vi "Autopatch-v2.1.vi"() -> ()   [LabVIEW 2016]
uses:
  <vilib>/userdefined/High Color/IMAQdx.ctl
  <vilib>/DAQmx/write.llb/DAQmx Write (Analog DBL 1Chan 1Samp).vi
  <vilib>/DAQmx/write.llb/DAQmx Write (Analog Wfm 1Chan NSamp).vi
  <vilib>/DAQmx/read.llb/DAQmx Read (Analog Wfm 1Chan NSamp).vi
  <vilib>/Analysis/baseanly.llb/Mean (DBL).vi
  <vilib>/DAQmx/create/channels.llb/DAQmx Create Channel (AO-Voltage-Basic).vi
  <vilib>/DAQmx/miscellaneous.llb/DAQmx Fill In Error Info.vi
  <vilib>/DAQmx/create/channels.llb/DAQmx Create Channel (AI-Voltage-Basic).vi
  <vilib>/DAQmx/configure/timing.llb/DAQmx Timing (Sample Clock).vi
  <vilib>/DAQmx/configure/trigger.llb/DAQmx Start Trigger (Digital Edge).vi
  <vilib>/Waveform/WDTOps.llb/WDT Waveform Duration DBL.vi
  <vilib>/addons/control/pid/pid.llb/PID (DBL).vi
  <vilib>/vision/driver/NI_Vision_Acquisition_Software.lvlib
  <resource>/objmgr/daqmx.rc
  <vilib>/Analysis/NI_AALBase.lvlib
  <vilib>/measure/NI_MABase.lvlib
  <vilib>/vision/NI_Vision_Development_Module.lvlib
  <vilib>/addons/control/pid/NI_PID_pid.lvlib
  vs/cell/Debug/cell.dll
panel:
  in  "下降/向右":bool
  in  "down":bool
  in  "up":bool
  out "读取缓冲区":string
  in  "调焦步伐/um":i64(ring)=3 items=["1", "10", "100", "1000", "10000"]
  in  "停止运动":bool
  in  "设置移动步长":bool
  in  "返回Z轴坐标":bool
  out "x*y":dbl
  out "电阻值":dbl
  in  "钳制电位":i16(ring) items=["0mv", "-70mv"]
  out "数值":dbl
  in  "自动破膜":bool
  in  "控制箱刺激ON\n/放大器刺激":bool=TRUE
  out "cout":i32
  out "Image 3":T1(plugin-control)
  out "Image 2":T1(plugin-control)
  in  "对比图":bool
  in  "自动封接":bool
  in  "保存数据":bool
  out "是否匹配到？":bool
  in  "PID gains":T2={"proportional gain (Kc)"=-0.05, "integral time (Ti, min)"=0.0, "derivative time (Td, min)"=0.0} caption="PID增益" {"derivative time (Td, min)" format="%.3f"; "integral time (Ti, min)" format="%.3f"; "proportional gain (Kc)" format="%.3f"}
  in  "PID gains 2":T2={"proportional gain (Kc)"=0.05, "integral time (Ti, min)"=0.0, "derivative time (Td, min)"=0.0} caption="PID增益" {"derivative time (Td, min)" format="%.3f"; "integral time (Ti, min)" format="%.3f"; "proportional gain (Kc)" format="%.3f"}
  out "x+y 2":i16
  out "调焦值2":dbl
  out "调焦值 3":dbl
  out "调焦值 4":dbl
  out "变量":dbl
  out "布尔":bool
  in  "聚焦值数组":dbl[](array[numeric])
  in  "下降步伐/um":dbl=1.0
  in  "自动接触":bool
  out "清晰度评价函数":dbl(graph)
  in  "针尖自动移动":bool
  in  "针尖细对焦":bool
  in  "针尖粗对焦":bool
  out "二值化":T1(plugin-control)
  in  "Range":cluster{"Lower value":sgl, "Upper value":sgl}={"Lower value"=0.0, "Upper value"=150.0} {"Upper value" format="%.2f"; "Lower value" format="%.2f"}
  in  "Operation":T3(ring)=enum."Dilate"
  in  "Number of Erosion":i32=10
  out "Particle Reports (Pixels)":T4(array[cluster]) {"Orientation" format="%.2f"; "Dimensions"."Height" format="%.2f"; "Dimensions"."Width" format="%.2f"; "Center of Mass"."Y" format="%.2f"; "Center of Mass"."X" format="%.2f"; "Bounding Rect"."Bottom" format="%.2f"; "Bounding Rect"."Right" format="%.2f"; "Bounding Rect"."Top" format="%.2f"; "Bounding Rect"."Left" format="%.2f"; "Number of Holes" format="%.2f"; "Area" format="%.2f"}
  out "Right":dbl
  out "目标坐标":i32[](array[numeric])
  in  "针尖模板匹配":bool=TRUE
  in  "基路径":path=path "E:/膜片/膜片钳/程序/CCD/模板40倍.jpg"
  out "Number of Matches":i32
  in  "Minimum Contrast":i32 min=0 max=255 step=1
  in  "Minimum Match Score":sgl=650.0 min=0 max=1000 format="%.2f"
  in  "Number of Matches Requested":i32=1 min=1
  out "Matches 2":T5(array[cluster]) {"Bounding Box"."y" format="%.2f"; "Bounding Box"."x" format="%.2f"; "Position"."y" format="%.2f"; "Position"."x" format="%.2f"; "Score" format="%.2f"; "Scale" format="%.2f"; "Angle" format="%.2f"}
  in  "Match Mode":u16(ring) items=["Shift Invariant", "Rotation Invariant"]
  out "针尖坐标":sgl[](array[numeric])
  in  "入液阻值校准":bool
  out "校准的入液阻值":dbl
  out "错误输出 3":errorcluster caption="错误输出"
  in  "低负开关":bool
  in  "低正开关":bool
  in  "大气压":bool
  in  "高负开关":bool
  in  "高正开关":bool
  in  "case":dbl
  out "测量值":dbl
  out "给定值":dbl
  out "输出气压波形图表":cluster{dbl, "低负":dbl}(graph)
  in  "低负":sgl(knob)=-0.45548448
  in  "高负":sgl(knob)=-5.0
  in  "低正":sgl(knob)=0.49642125 scale=0.0..2.0
  in  "高正":sgl(knob)=10.718505 scale=0.0..15.0
  in  "采样率":u32=255
  in  "DevIndex":i32
  in  "Holding Voltage":dbl=-70.0
  out "Negative Peak":dbl
  out "阻值波形图表":dbl(graph)
  out "Resistance(MΩ)":dbl
  out "！":bool
  in  "下拉列表":u16(ring) items=["Voltage Clamp", "Current Clamp"]
  out "电流信号波形图":waveform(dbl)(graph)
  in  "frequency":dbl=20.0
  in  "Averaging":i32=5
  in  "amplitude":dbl=0.01
  in  "阻值数组":dbl[](array[numeric])
  out "循环时间":u32
  out "Image":T1(plugin-control)
  out "错误输出":errorcluster
  in  "停止":bool
  in  "Session In":T6="cam1"
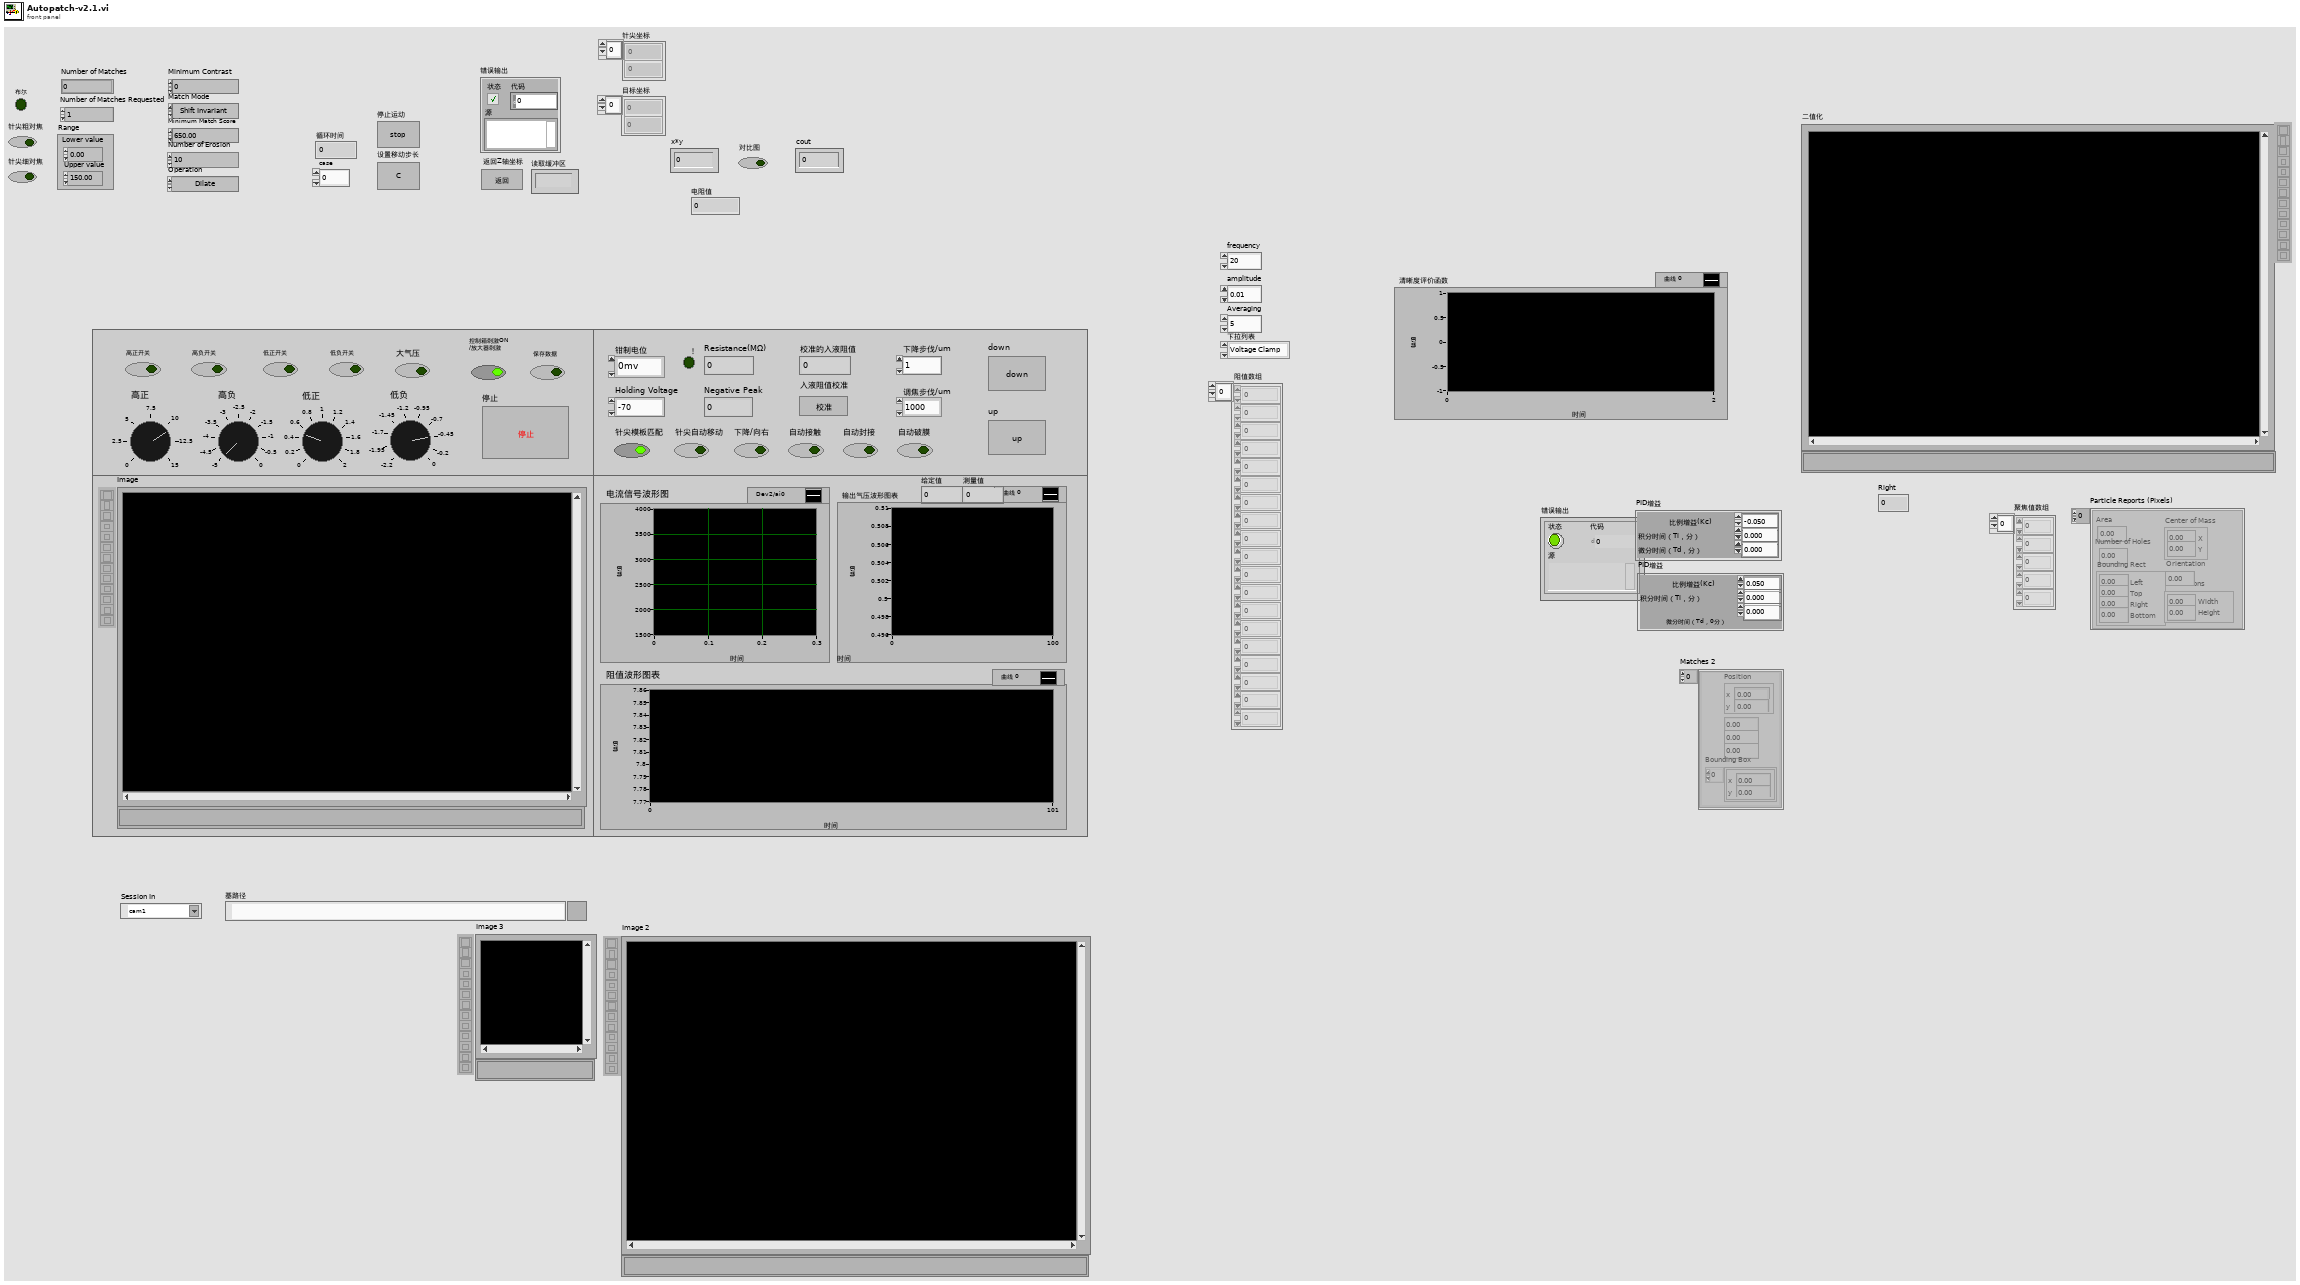
[diagram p1: front panel]
types:
  T1 = typedef "IMAQ Image.ctl" = refnum<image>
  T2 = cluster{"proportional gain (Kc)":dbl, "integral time (Ti, min)":dbl, "derivative time (Td, min)":dbl}
  T3 = enum32{"AutoM", "Close", "Dilate", "Erode", "Gradient", "Gradient out", "Gradient in", "Hit miss", "Open", "PClose", "POpen", "Thick", "Thin"}
  T4 = cluster{"Area":dbl, "Number of Holes":dbl, "Bounding Rect":cluster{"Left":dbl, "Top":dbl, "Right":dbl, "Bottom":dbl}, "Center of Mass":cluster{"X":dbl, "Y":dbl}, "Orientation":dbl, "Dimensions":cluster{"Width":dbl, "Height":dbl}}[]
  T5 = cluster{"Position":cluster{"x":sgl, "y":sgl}, "Angle":sgl, "Scale":sgl, "Score":sgl, "Bounding Box":cluster{"x":sgl, "y":sgl}[]}[]
  T6 = typedef "IMAQdx.ctl" = refnum<k21>
  T7 = enum16{"open", "replace", "create", "open or create", "replace or create", "replace or create with confirmation"}
  T8 = typedef "Image Type" = u32
  T9 = cluster{"Averaging":i32, "frequency":dbl, "amplitude":dbl, "Proportion":dbl, "Fs":dbl}
  T10 = enum16{"Sine Wave", "Triangle Wave", "Square Wave", "Sawtooth Wave"}
  T11 = cluster{"Global Rectangle":i32[], "Contours":cluster{"Contour Type":u32, "ROI Type":u32, "Points":i32[]}[]}
  T12 = cluster{"Position":cluster{"x":sgl, "y":sgl}, "Angle":sgl, "Scale":sgl, "Score":sgl, "Bounding Box":cluster{"x":sgl, "y":sgl}[]}
  T13 = cluster{"Area":dbl, "Number of Holes":dbl, "Bounding Rect":cluster{"Left":dbl, "Top":dbl, "Right":dbl, "Bottom":dbl}, "Center of Mass":cluster{"X":dbl, "Y":dbl}, "Orientation":dbl, "Dimensions":cluster{"Width":dbl, "Height":dbl}}
  T14 = cluster{"Left":dbl, "Top":dbl, "Right":dbl, "Bottom":dbl}
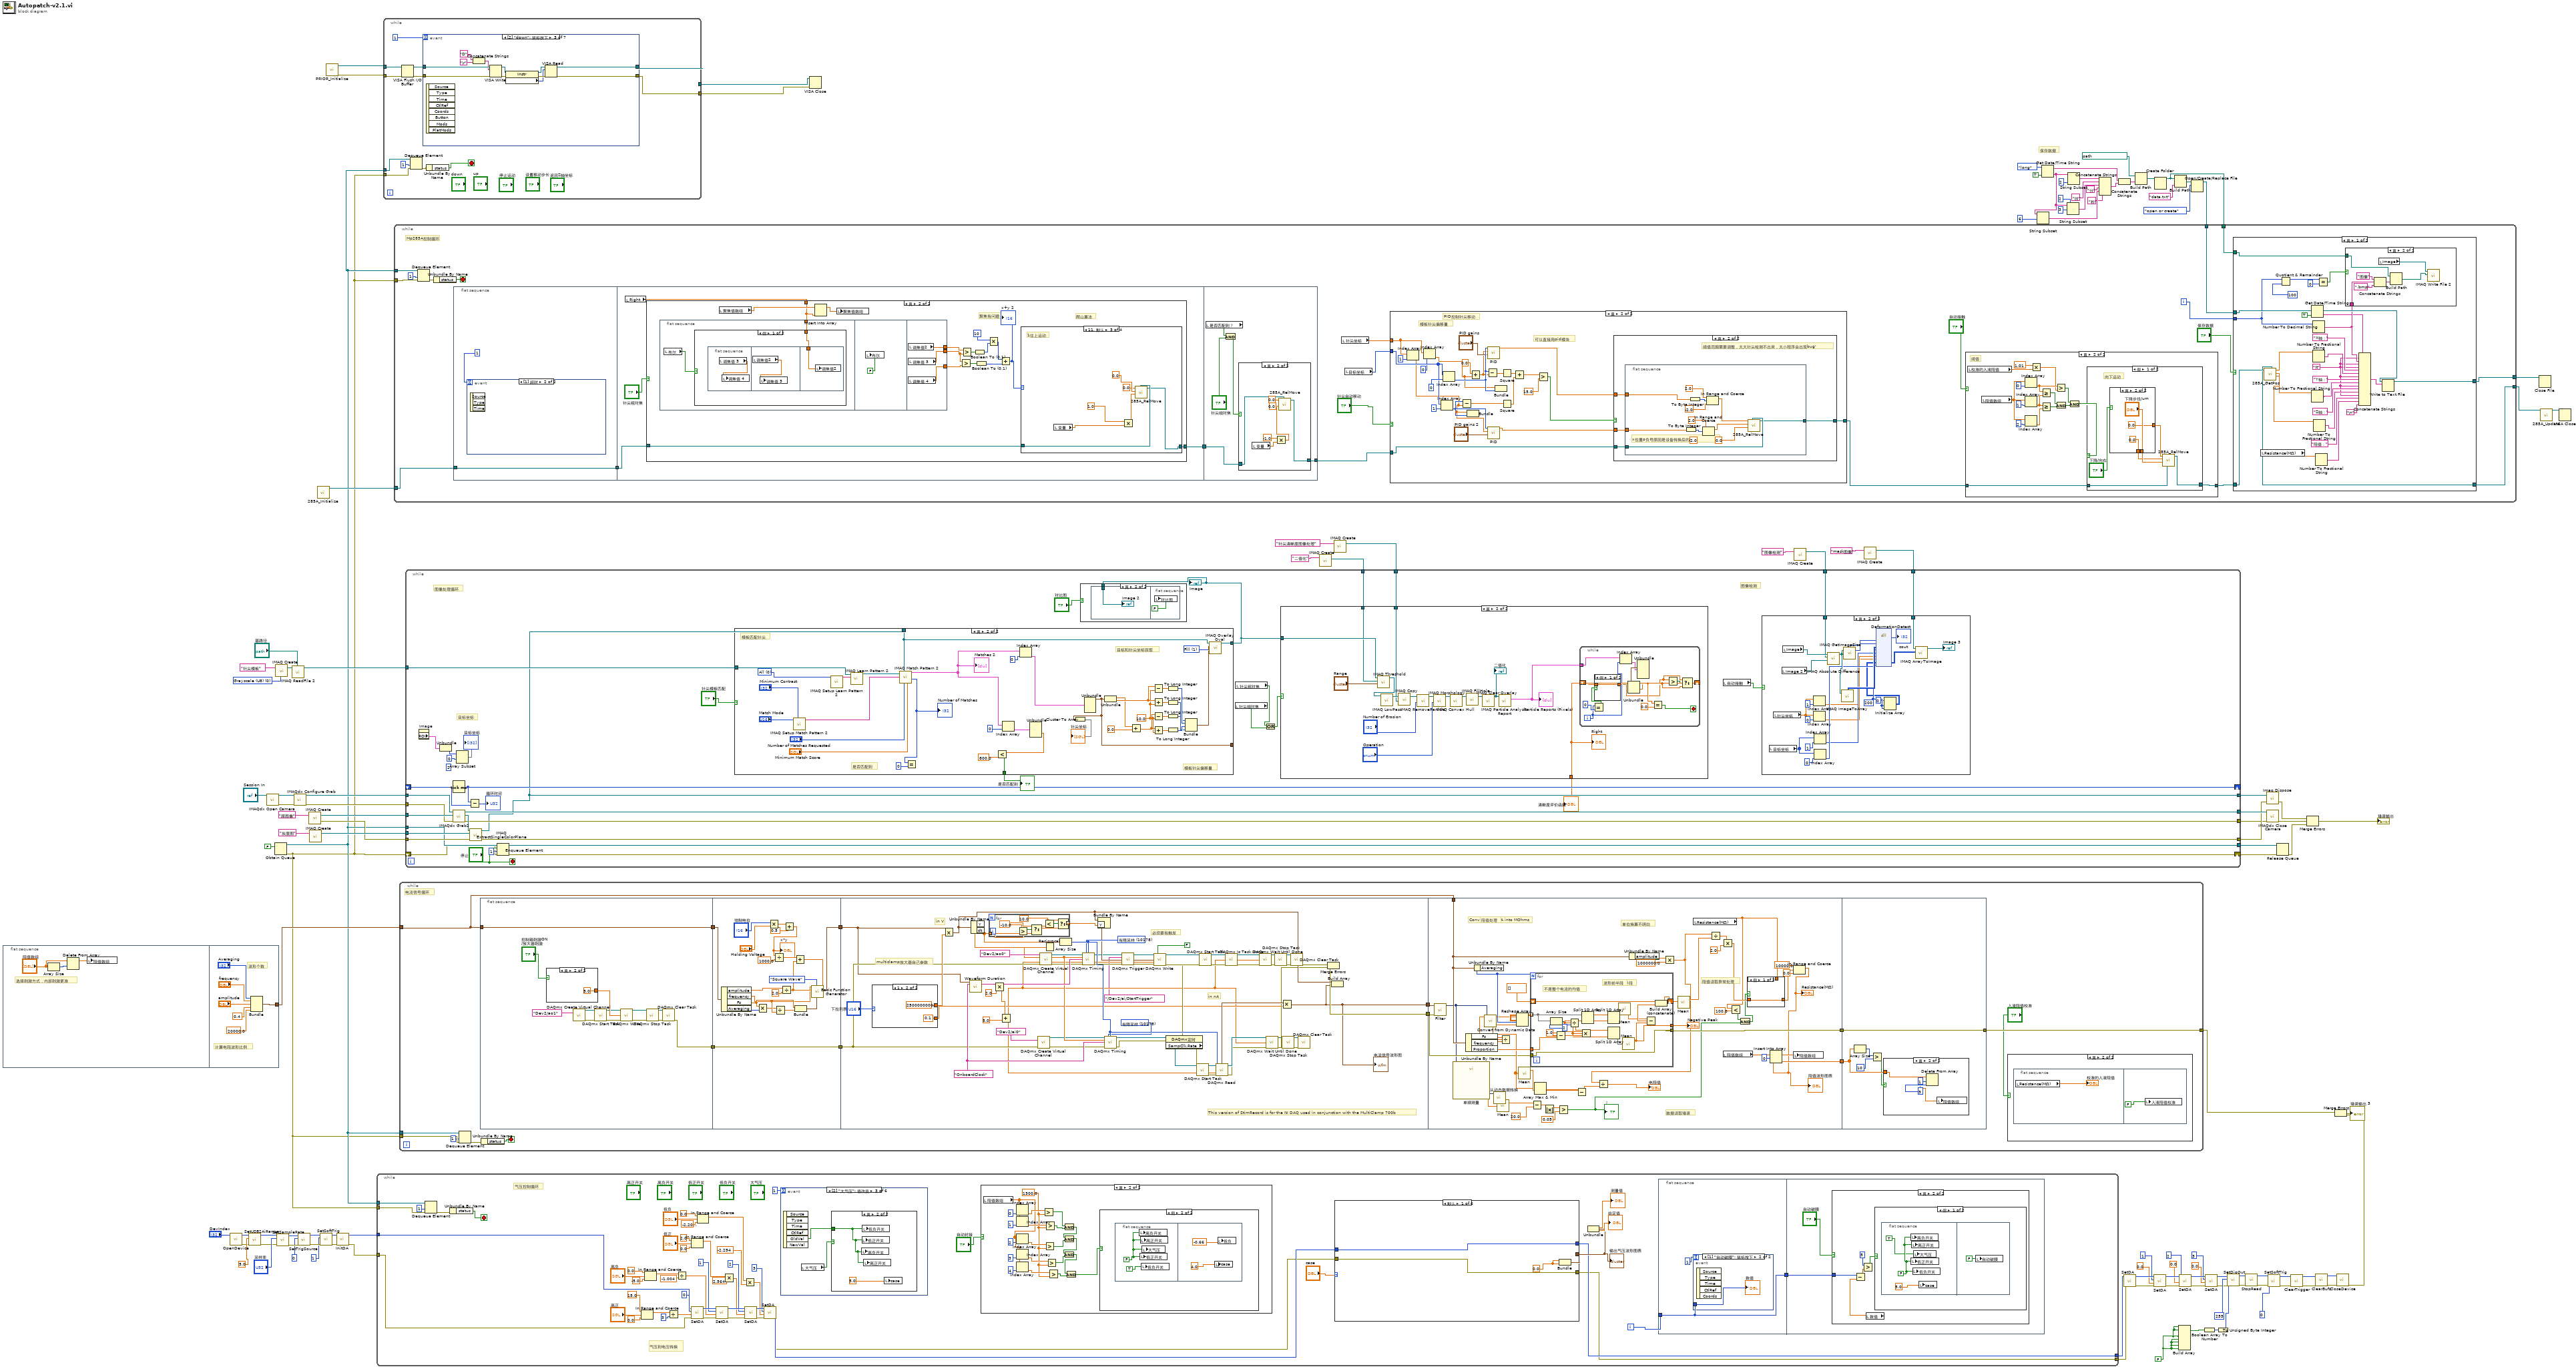
[diagram p0: block diagram]
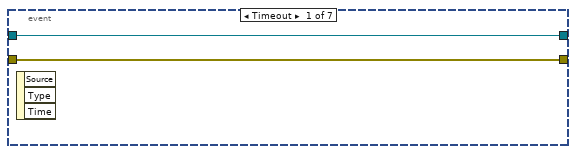
[diagram p2: hidden frame]
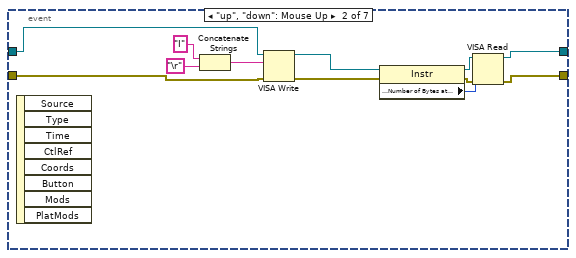
[diagram p3: hidden frame]
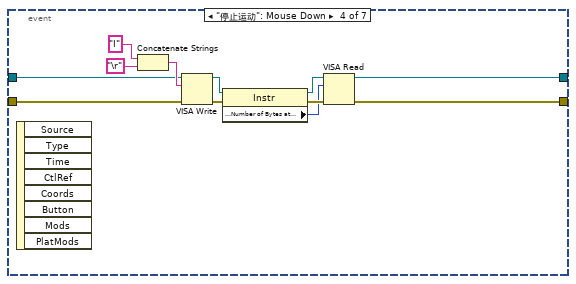
[diagram p4: hidden frame]
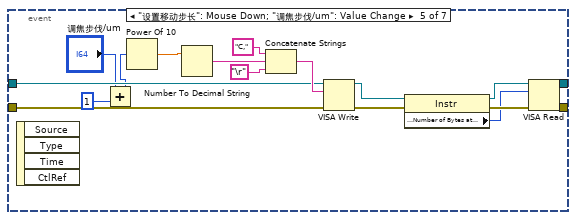
[diagram p5: hidden frame]
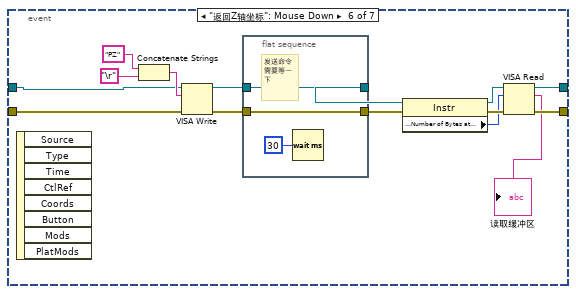
[diagram p6: hidden frame]
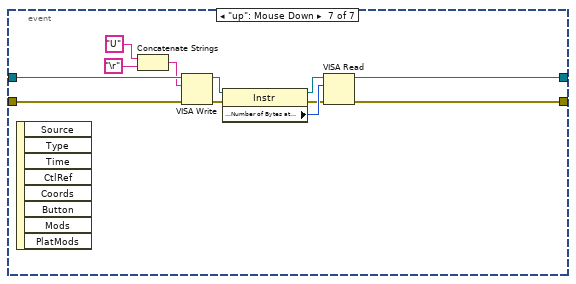
[diagram p7: hidden frame]
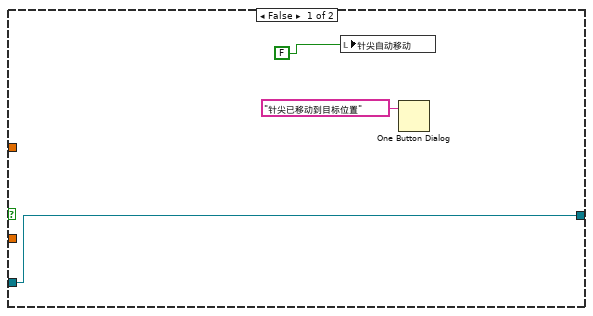
[diagram p11: hidden frame]
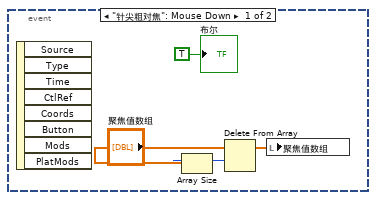
[diagram p12: hidden frame]
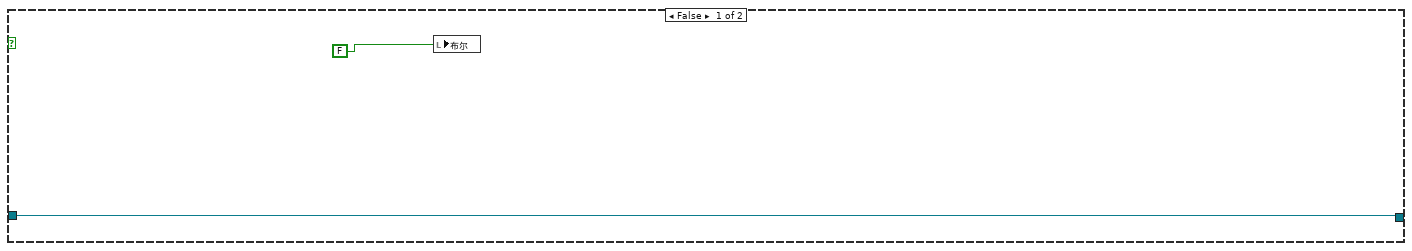
[diagram p13: hidden frame]
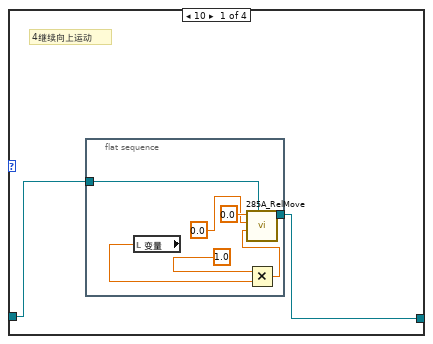
[diagram p14: hidden frame]
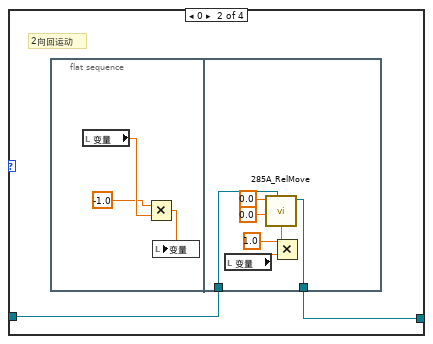
[diagram p15: hidden frame]
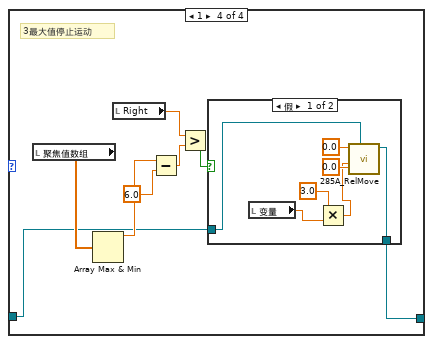
[diagram p16: hidden frame]
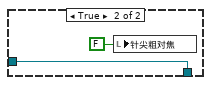
[diagram p17: hidden frame]
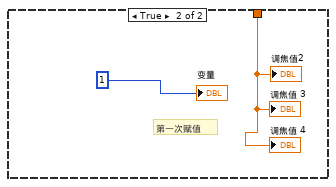
[diagram p18: hidden frame]
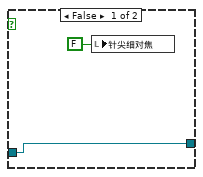
[diagram p19: hidden frame]
diagram:
  w47 = T8 0 items=["Grayscale (U8)", "Grayscale (I16)", "Grayscale (SGL)", "Complex (CSG)", "RGB (U32)", "HSL (U32)", "RGB (U64)", "Grayscale (U16)"] ("Image Type")
  w61 = FALSE
  # "保存数据"
  n1 = flat-sequence {
    tunnel: [w124] -> w108
    frame #0 {
      # "选择刺激方式，内部刺激更准"
      n2 = Array Size(array="阻值数组") -> (size(s)=w123:i32)
      n3 = Delete From Array(array="阻值数组", length=w123) -> (array with subset deleted=w121:dbl[])  [unwired: 1 in, 1 out]
      n4 = local write "阻值数组"(w121) -> ()
    }
    frame #1 {
      # "波形个数"
      # "计算电阻波形比例"
      n5 = Bundle("Averaging"="Averaging", "frequency"="frequency", "amplitude"="amplitude", "Proportion"=0.4, "Fs"=20000.0) -> (w124:T9)  [unwired: 1 in]
    }
  }
  n6 = call "OpenDevice.vi"("DevIndex"="DevIndex") -> ("错误输出"=w88:errorcluster, "DevIndex Output"=w86:i32)  [unwired: 9 in]
  n7 = call "SetUSB2AiRange.vi"("错误输入（无错误）"=w88, "Range"=sgl 5.0, "DevIndex"=w86) -> ("错误输出"=w97:errorcluster, "DevIndex Output"=w95:i32)  [unwired: 7 in]
  n8 = call <vilib>:"IMAQdx Open Camera.vi"("Session In"="Session In") -> ("error out"=w120:errorcluster, "Session Out"=w117:T6)  [unwired: 9 in]
  n9 = Obtain Queue(element data type=FALSE) -> (queue out=w2:refnum<queue>, error out=w1:errorcluster)  [unwired: 4 in, 1 out]
  n10 = call "IMAQ Create"("Image Name"="针尖模板", "Image Type"=w47) -> ("New Image"=w48:T1)  [unwired: 3 in, 1 out]
  n11 = call "SetSampleRate.vi"("错误输入（无错误）"=w97, "SampleRate"="采样率", "DevIndex"=w95) -> ("错误输出"=w98:errorcluster, "DevIndex Output"=w96:i32)  [unwired: 7 in]
  n12 = call "IMAQ ReadFile 2"("File Path"="基路径", "Image"=w48) -> ("Image Out"=w46:T1)  [unwired: 5 in, 4 out]
  n13 = call <vilib>:"IMAQdx Configure Grab.vi"("error in"=w120, "Session In"=w117) -> ("error out"=w105:errorcluster, "Session Out"=w118:T6)  [unwired: 8 in]
  n14 = call "SetTrigSource.vi"("错误输入（无错误）"=w98, "TrigSource"=u8 0, "DevIndex"=w96) -> ("错误输出"=w93:errorcluster, "DevIndex Output"=w92:i32)  [unwired: 7 in]
  n15 = call "IMAQ Create"("Image Name"="原图像") -> ("New Image"=w116:T1, "error out"=w103:errorcluster)  [unwired: 4 in]
  n16 = call "IMAQ Create"("Image Name"="灰度图") -> ("New Image"=w109:T1)  [unwired: 4 in, 1 out]
  n17 = call "285A_Initialize.vi"() -> ("VISA资源名称输出"=w41:refnum<visa-resource-name>)  [unwired: 10 in, 1 out]
  n18 = call "SetSoftTrig.vi"("错误输入（无错误）"=w93, "Trig"=u8 1, "DevIndex"=w92) -> ("错误输出"=w89:errorcluster, "DevIndex Output"=w87:i32)  [unwired: 7 in]
  n19 = call "PRIOR_Initialize.vi"() -> ("错误输出"=w5:errorcluster, "VISA资源名称输出"=w6:refnum<visa-resource-name>)  [unwired: 10 in]
  n20 = call "InitDA.vi"("错误输入（无错误）"=w89, "DevIndex"=w87) -> ("错误输出"=w83:errorcluster, "DevIndex Output"=w84:i32)  [unwired: 8 in]
  n21 = while {
    tunnel: w84 -> [w143]
    tunnel: w2 -> [w182]
    tunnel: w1 -> [w181]
    tunnel: [w135] -> w8
    tunnel: w83 -> [w142]
    tunnel: [w133] -> w7
    i -> [w131]
    stop <- w178 stop-if-true
    # "气压控制循环"
    # "气压到电压转换"
    n22 = Dequeue Element(queue=w182, timeout in ms (-1)=1 ("超时毫秒(-1)"), error in (no error)=w181) -> (error out=w179:errorcluster)  [unwired: 3 out]
    n23 = Unbundle By Name(w179) -> ("status"=w178:bool)
    n24 = In Range and Coerce(upper limit=sgl 15.0 ("上限"), x="高正", lower limit=sgl 0.0 ("下限")) -> (coerced(x)=w146:sgl)  [unwired: 1 out]
    n25 = In Range and Coerce(upper limit=sgl 0.0 ("上限"), x="高负", lower limit=sgl -5.0 ("下限")) -> (coerced(x)=w150:sgl)  [unwired: 1 out]
    n26 = Divide(x=w146, y=3) -> (x/y=w167:sgl)
    n27 = Divide(x=w150, y=-1.004) -> (x/y=w163:dbl)
    n28 = In Range and Coerce(upper limit=sgl 2.0 ("上限"), x="低正", lower limit=sgl 0.0 ("下限")) -> (coerced(x)=w154:sgl)  [unwired: 1 out]
    n29 = call "SetDA.vi"("错误输入（无错误）"=w142, "DAVolt"=w167, "DANum"=u8 0, "DevIndex"=w143) -> ("错误输出"=w176:errorcluster, "DevIndex Output"=w177:i32)  [unwired: 6 in]
    n30 = In Range and Coerce(upper limit=sgl 0.0 ("上限"), x="低负", lower limit=sgl -2.2 ("下限")) -> (coerced(x)=w156:sgl)  [unwired: 1 out]
    n31 = call "SetDA.vi"("错误输入（无错误）"=w176, "DAVolt"=w163, "DANum"=u8 1, "DevIndex"=w177) -> ("错误输出"=w175:errorcluster, "DevIndex Output"=w174:i32)  [unwired: 6 in]
    n32 = Multiply(x=w154, y=2.564) -> (x*y=w160:dbl)
    n33 = Multiply(x=w156, y=-2.294) -> (x*y=w161:dbl)
    n34 = call "SetDA.vi"("错误输入（无错误）"=w175, "DAVolt"=w160, "DANum"=u8 2, "DevIndex"=w174) -> ("错误输出"=w172:errorcluster, "DevIndex Output"=w173:i32)  [unwired: 6 in]
    n35 = call "SetDA.vi"("错误输入（无错误）"=w172, "DAVolt"=w161, "DANum"=u8 3, "DevIndex"=w173) -> ("错误输出"=w136:errorcluster, "DevIndex Output"=w137:i32)  [unwired: 6 in]
    n36 = event shown="[2] \"大气压\": 值改变" {
      selector: _ -> [_ _ _ _ _ _]
      dyn-events: _ -> [_ _ _ _ _ _]
      timeout: 1 -> [_ _ _ _ _ _]
      event "高正开关": Value Change {
        n37 = event-data() -> ("OldVal"=w231:bool)  [unwired: 1 in, 5 out]
        n38 = local read "高正开关"() -> (w232:bool)
        n39 = case shown="真" w232 {
          tunnel: w231 -> [_ w234]
          frame False {
          }
          frame True {
            n40 = local write "高负开关"(w234) -> ()
            n41 = local write "低负开关"(w234) -> ()
            n42 = local write "低正开关"(w234) -> ()
            n43 = local write "大气压"(w234) -> ()
            n44 = local write "case"(1.0) -> ()
          }
        }
      }
      event Timeout {
        n45 = event-data() -> ()  [unwired: 1 in, 3 out]
      }
      event "大气压": Value Change {
        n46 = event-data() -> ("OldVal"=w235:bool)  [unwired: 1 in, 5 out]
        n47 = local read "大气压"() -> (w236:bool)
        n48 = case shown="真" w236 {
          tunnel: w235 -> [_ w238]
          frame False {
          }
          frame True {
            n49 = local write "高负开关"(w238) -> ()
            n50 = local write "低正开关"(w238) -> ()
            n51 = local write "低负开关"(w238) -> ()
            n52 = local write "高正开关"(w238) -> ()
            n53 = local write "case"(5.0) -> ()
          }
        }
      }
      event "低正开关": Value Change {
        n54 = event-data() -> ("OldVal"=w240:bool)  [unwired: 1 in, 5 out]
        n55 = local read "低正开关"() -> (w239:bool)
        n56 = case shown="真" w239 {
          tunnel: w240 -> [_ w242]
          frame False {
          }
          frame True {
            n57 = local write "高正开关"(w242) -> ()
            n58 = local write "高负开关"(w242) -> ()
            n59 = local write "低负开关"(w242) -> ()
            n60 = local write "大气压"(w242) -> ()
            n61 = local write "case"(3.0) -> ()
          }
        }
      }
      event "低负开关": Value Change {
        n62 = event-data() -> ("OldVal"=w244:bool)  [unwired: 1 in, 5 out]
        n63 = local read "低负开关"() -> (w243:bool)
        n64 = case shown="真" w243 {
          tunnel: w244 -> [_ w246]
          frame False {
          }
          frame True {
            n65 = local write "高负开关"(w246) -> ()
            n66 = local write "低正开关"(w246) -> ()
            n67 = local write "高正开关"(w246) -> ()
            n68 = local write "大气压"(w246) -> ()
            n69 = local write "case"(4.0) -> ()
          }
        }
      }
      event "高负开关": Value Change {
        n70 = event-data() -> ("OldVal"=w248:bool)  [unwired: 1 in, 5 out]
        n71 = local read "高负开关"() -> (w247:bool)
        n72 = case shown="真" w247 {
          tunnel: w248 -> [_ w250]
          frame False {
          }
          frame True {
            n73 = local write "低正开关"(w250) -> ()
            n74 = local write "低负开关"(w250) -> ()
            n75 = local write "高正开关"(w250) -> ()
            n76 = local write "大气压"(w250) -> ()
            n77 = local write "case"(2.0) -> ()
          }
        }
      }
    }
    n78 = case shown="真" "自动封接" {
      frame False {
      }
      frame True {
        w205 = 1300.0 ("y")
        n79 = local read "阻值数组"() -> (w206:dbl[])
        n80 = Index Array(array=w206, index=0 ("索引")) -> (element=w208:dbl)
        n81 = Index Array(array=w206, index=1 ("索引")) -> (element=w207:dbl)
        n82 = Index Array(array=w206, index=2 ("索引")) -> (element=w216:dbl)
        n83 = Index Array(array=w206, index=3 ("索引")) -> (element=w215:dbl)
        n84 = Index Array(array=w206, index=4 ("索引")) -> (element=w214:dbl)
        n85 = Greater?(x=w208, y=w205) -> (0:w213:bool)
        n86 = Greater?(x=w216, y=w205) -> (0:w211:bool)
        n87 = Greater?(x=w207, y=w205) -> (0:w212:bool)
        n88 = Greater?(x=w215, y=w205) -> (0:w210:bool)
        n89 = Greater?(x=w214, y=w205) -> (0:w209:bool)
        n90 = And(x=w213, y=w212) -> (x .and. y?=w204:bool)
        n91 = And(x=w204, y=w211) -> (x .and. y?=w203:bool)
        n92 = And(x=w203, y=w210) -> (x .and. y?=w202:bool)
        n93 = And(x=w202, y=w209) -> (x .and. y?=w201:bool)
        n94 = case shown="假" w201 {
          frame True {
            n95 = flat-sequence {
              frame #0 {
                w222 = FALSE
                n96 = local write "高负开关"(w222) -> ()
                n97 = local write "低负开关"(w222) -> ()
                n98 = local write "低正开关"(w222) -> ()
                n99 = local write "高正开关"(w222) -> ()
                n100 = local write "大气压"(TRUE) -> ()
              }
              frame #1 {
                n101 = local write "case"(5.0) -> ()
              }
              frame #2 {
                n102 = local write "自动封接"(FALSE) -> ()
                n103 = One Button Dialog(message="已形成G欧封接！" ("消息")) -> ()  [unwired: 1 in, 1 out]
              }
            }
          }
          frame False {
            n104 = flat-sequence {
              frame #0 {
                w227 = FALSE
                n105 = local write "高负开关"(w227) -> ()
                n106 = local write "低正开关"(w227) -> ()
                n107 = local write "高正开关"(w227) -> ()
                n108 = local write "低负开关"(TRUE) -> ()
                n109 = local write "大气压"(w227) -> ()
              }
              frame #1 {
                n110 = local write "case"(4.0) -> ()
                n111 = local write "低负"(-0.66) -> ()
              }
            }
          }
        }
      }
    }
    n112 = case shown="默认" "case" {
      tunnel: w137 -> [w254 w274 w296 w320 w344 w357]
      tunnel: w136 -> [w253 w273 w295 w319 w343 w356]
      tunnel: [w254 w256 w287 w314 w336 w354] -> w135
      tunnel: [w253 w264 w288 w313 w337 w353] -> w133
      tunnel: [w251 w255 w279 w303 w327 w351] -> w139
      frame Default {
        w252 = 0.0
        n113 = Bundle(w252, w252) -> (w251:cluster{dbl, dbl})  [unwired: 1 in]
      }
      frame 1 {
        w271 = TRUE
        w272 = FALSE
        n114 = Build Array(w272, w271, w271, w272, w272, w272, w272, w272) -> (w275:bool[])
        n115 = Boolean Array To Number(Boolean array=w275) -> (number=w278:u32)
        n116 = To Unsigned Byte Integer(number=w278) -> (unsigned 8bit integer=w277:u8)
        n117 = call "StartRead.vi"("错误输入（无错误）"=w273, "DevIndex"=w274) -> ("错误输出"=w269:errorcluster, "DevIndex Output"=w270:i32)  [unwired: 8 in]
        n118 = call "SetDioOut.vi"("错误输入（无错误）"=w269, "DioOut"=w277, "DioChanSel"=u8 255, "DevIndex"=w270) -> ("错误输出"=w265:errorcluster, "DevIndex Output"=w266:i32)  [unwired: 6 in]
        n119 = call "GetAiChans.vi"("错误输入（无错误）"=w265, "Num"=u32 1, "ChanSel"=u16 1, "DevIndex"=w266) -> ("错误输出"=w264:errorcluster, "Ai"=w261:sgl[][], "DevIndex Output"=w256:i32)  [unwired: 4 in, 1 out]
        n120 = Index Array(array=w261, index (row)=0, index (col)=0) -> (element=w258:sgl)
        n121 = local read "高正"() -> (w260:sgl)
        n122 = Multiply(x=w258, y=3) -> (x*y=w257:sgl)
        n123 = Bundle(w257, "高正"=w260) -> (w255:cluster{sgl, "高正":sgl})  [unwired: 1 in]
      }
      frame 2 {
        w294 = TRUE
        w293 = FALSE
        n124 = Build Array(w293, w294, w293, w293, w294, w293, w293, w293) -> (w297:bool[])
        n125 = Boolean Array To Number(Boolean array=w297) -> (number=w302:u32)
        n126 = To Unsigned Byte Integer(number=w302) -> (unsigned 8bit integer=w301:u8)
        n127 = call "StartRead.vi"("错误输入（无错误）"=w295, "DevIndex"=w296) -> ("错误输出"=w298:errorcluster, "DevIndex Output"=w299:i32)  [unwired: 8 in]
        n128 = call "SetDioOut.vi"("错误输入（无错误）"=w298, "DioOut"=w301, "DioChanSel"=u8 255, "DevIndex"=w299) -> ("错误输出"=w289:errorcluster, "DevIndex Output"=w290:i32)  [unwired: 6 in]
        n129 = call "GetAiChans.vi"("错误输入（无错误）"=w289, "Num"=u32 1, "ChanSel"=u16 2, "DevIndex"=w290) -> ("错误输出"=w288:errorcluster, "Ai"=w284:sgl[][], "DevIndex Output"=w287:i32)  [unwired: 4 in, 1 out]
        n130 = Unbundle(w289) -> ()  [unwired: 3 out]
        n131 = Index Array(array=w284, index (row)=0, index (col)=0) -> (element=w282:sgl)
        n132 = local read "高负"() -> (w283:sgl)
        n133 = Multiply(x=w282, y=-1.004) -> (x*y=w280:dbl)
        n134 = Bundle(w280, "高负"=w283) -> (w279:cluster{dbl, "高负":sgl})  [unwired: 1 in]
      }
      frame 3 {
        w305 = FALSE
        n135 = Build Array(w305, w305, w305, TRUE, w305, w305, w305, w305) -> (w321:bool[])
        n136 = Boolean Array To Number(Boolean array=w321) -> (number=w326:u32)
        n137 = To Unsigned Byte Integer(number=w326) -> (unsigned 8bit integer=w325:u8)
        n138 = call "StartRead.vi"("错误输入（无错误）"=w319, "DevIndex"=w320) -> ("错误输出"=w322:errorcluster, "DevIndex Output"=w323:i32)  [unwired: 8 in]
        n139 = call "SetDioOut.vi"("错误输入（无错误）"=w322, "DioOut"=w325, "DioChanSel"=u8 255, "DevIndex"=w323) -> ("错误输出"=w315:errorcluster, "DevIndex Output"=w316:i32)  [unwired: 6 in]
        n140 = call "GetAiChans.vi"("错误输入（无错误）"=w315, "Num"=u32 1, "ChanSel"=u16 4, "DevIndex"=w316) -> ("错误输出"=w313:errorcluster, "Ai"=w310:sgl[][], "DevIndex Output"=w314:i32)  [unwired: 4 in, 1 out]
        n141 = Unbundle(w315) -> ()  [unwired: 3 out]
        n142 = Index Array(array=w310, index (row)=0, index (col)=0) -> (element=w308:sgl)
        n143 = local read "低正"() -> (w309:sgl)
        n144 = Divide(x=w308, y=2.564) -> (x/y=w306:dbl)
        n145 = Bundle(w306, "低正"=w309) -> (w303:cluster{dbl, "低正":sgl})  [unwired: 1 in]
      }
      frame 4 {
        w328 = FALSE
        n146 = call "StartRead.vi"("错误输入（无错误）"=w343, "DevIndex"=w344) -> ("错误输出"=w346:errorcluster, "DevIndex Output"=w347:i32)  [unwired: 8 in]
        n147 = local read "低负"() -> (w332:sgl)
        n148 = Build Array(w328, w328, w328, w328, w328, TRUE, w328, w328) -> (w345:bool[])
        n149 = Boolean Array To Number(Boolean array=w345) -> (number=w350:u32)
        n150 = To Unsigned Byte Integer(number=w350) -> (unsigned 8bit integer=w349:u8)
        n151 = call "SetDioOut.vi"("错误输入（无错误）"=w346, "DioOut"=w349, "DioChanSel"=u8 255, "DevIndex"=w347) -> ("错误输出"=w338:errorcluster, "DevIndex Output"=w339:i32)  [unwired: 6 in]
        n152 = Unbundle(w338) -> ()  [unwired: 3 out]
        n153 = call "GetAiChans.vi"("错误输入（无错误）"=w338, "Num"=u32 1, "ChanSel"=u16 8, "DevIndex"=w339) -> ("错误输出"=w337:errorcluster, "Ai"=w333:sgl[][], "DevIndex Output"=w336:i32)  [unwired: 4 in, 1 out]
        n154 = Index Array(array=w333, index (row)=0, index (col)=0) -> (element=w331:sgl)
        n155 = Divide(x=w331, y=-2.294) -> (x/y=w329:dbl)
        n156 = Bundle(w329, "低负"=w332) -> (w327:cluster{dbl, "低负":sgl})  [unwired: 1 in]
      }
      frame 5 {
        w352 = 0.0
        (unwired) TRUE
        w355 = FALSE
        n157 = call "StartRead.vi"("错误输入（无错误）"=w356, "DevIndex"=w357) -> ("错误输出"=w359:errorcluster, "DevIndex Output"=w360:i32)  [unwired: 8 in]
        n158 = Build Array(w355, w355, w355, w355, w355, w355, w355, w355) -> (w358:bool[])
        n159 = Boolean Array To Number(Boolean array=w358) -> (number=w363:u32)
        n160 = To Unsigned Byte Integer(number=w363) -> (unsigned 8bit integer=w362:u8)
        n161 = call "SetDioOut.vi"("错误输入（无错误）"=w359, "DioOut"=w362, "DioChanSel"=u8 255, "DevIndex"=w360) -> ("错误输出"=w353:errorcluster, "DevIndex Output"=w354:i32)  [unwired: 6 in]
        n162 = Unbundle(w353) -> ()  [unwired: 3 out]
        n163 = Bundle(w352, w352) -> (w351:cluster{dbl, dbl})  [unwired: 1 in]
      }
    }
    "输出气压波形图表" <- w139
    n164 = Unbundle(w139) -> (→"测量值":dbl, "高正"=→"给定值":dbl)
    n165 = flat-sequence {
      tunnel: w131 -> [w183]
      tunnel: [w183] -> w130
      tunnel: w130 -> [w186]
      frame #0 {
        n166 = event shown="[1] \"自动破膜\": 鼠标按下" {
          selector: _ -> [_ _]
          dyn-events: _ -> [_ _]
          timeout: 1 -> [_ _]
          tunnel: w183 -> [_ w185]
          event Timeout {
            n167 = event-data() -> ()  [unwired: 1 in, 3 out]
          }
          event "自动破膜": Mouse Down {
            n168 = event-data() -> ()  [unwired: 1 in, 5 out]
            "数值" <- w185
          }
        }
      }
      frame #1 {
        n169 = case shown="真" "自动破膜" {
          tunnel: w186 -> [_ w188]
          frame False {
          }
          frame True {
            n170 = local read "数值"() -> (w192:dbl)
            n171 = Subtract(x=w188, y=w192) -> (x-y=w190:dbl)
            n172 = Greater?(x=5, y=w190) -> (0:w191:bool)
            n173 = case shown="假" w191 {
              frame False {
                n174 = flat-sequence {
                  frame #0 {
                    w195 = FALSE
                    n175 = local write "高负开关"(w195) -> ()
                    n176 = local write "低正开关"(w195) -> ()
                    n177 = local write "高正开关"(w195) -> ()
                    n178 = local write "低负开关"(w195) -> ()
                    n179 = local write "大气压"(TRUE) -> ()
                    n180 = local write "case"(5.0) -> ()
                  }
                  frame #1 {
                    n181 = local write "自动破膜"(FALSE ("自动破膜")) -> ()
                  }
                }
              }
              frame True {
                n182 = flat-sequence {
                  frame #0 {
                    w199 = FALSE
                    n183 = local write "高负开关"(TRUE) -> ()
                    n184 = local write "低正开关"(w199) -> ()
                    n185 = local write "高正开关"(w199) -> ()
                    n186 = local write "低负开关"(w199) -> ()
                    n187 = local write "大气压"(w199) -> ()
                    n188 = local write "case"(2.0) -> ()
                  }
                  frame #1 {
                    n189 = local write "高负"(-5.0) -> ()
                  }
                }
              }
            }
          }
        }
      }
    }
  }
  n190 = while {
    tunnel: w5 -> [w372]
    tunnel: w6 -> [w373]
    tunnel: [w369] -> w3
    tunnel: [w374] -> w4
    tunnel: w2 -> [w366]
    tunnel: w1 -> [w365]
    stop <- w364 stop-if-true
    n191 = VISA Flush I/O Buffer(VISA resource name=w373, error in (no error)=w372) -> (VISA resource name out=w371:refnum<visa-resource-name>, error out=w370:errorcluster)  [unwired: 1 in]
    n192 = Dequeue Element(queue=w366, timeout in ms (-1)=1 ("超时毫秒(-1)"), error in (no error)=w365) -> (error out=w368:errorcluster)  [unwired: 3 out]
    n193 = event shown="[2] \"down\": 鼠标按下" {
      selector: _ -> [_ _ _ _ _ _ _]
      dyn-events: _ -> [_ _ _ _ _ _ _]
      timeout: 1 -> [_ _ _ _ _ _ _]
      tunnel: [w377 w379 w401 w403 w421 w437 w460] -> w374
      tunnel: [w376 w378 w400 w402 w420 w436 w459] -> w369
      tunnel: w371 -> [w377 w381 w399 w405 w423 w439 w458]
      tunnel: w370 -> [w376 w380 w398 w404 w422 w438 w457]
      event Timeout {
        n194 = event-data() -> ()  [unwired: 1 in, 3 out]
      }
      event "up", "down": Mouse Up {
        n195 = event-data() -> ()  [unwired: 1 in, 8 out]
        n196 = Concatenate Strings("I" ("写入缓冲区"), "\r") -> (w389:string)
        n197 = VISA Write ("VISA写入")(VISA resource name=w381, write buffer=w389, error in (no error)=w380) -> (VISA resource name out=w383:refnum<visa-resource-name>, error out=w382:errorcluster)  [unwired: 1 out]
        n198 = property class="Instr"(reference=w383, error in=w382) -> (reference out=w384:refnum<visa-resource-name>, error out=w385:errorcluster, "Serial Settings:Number of Bytes at Serial Port"=w386:u32)
        n199 = VISA Read(VISA resource name=w384, byte count=w386, error in (no error)=w385) -> (VISA resource name out=w379:refnum<visa-resource-name>, error out=w378:errorcluster)  [unwired: 2 out]
      }
      event "down": Mouse Down {
        n200 = event-data() -> ()  [unwired: 1 in, 8 out]
        n201 = Concatenate Strings("D" ("写入缓冲区"), "\r") -> (w390:string)
        n202 = VISA Write ("VISA写入")(VISA resource name=w399, write buffer=w390, error in (no error)=w398) -> (VISA resource name out=w396:refnum<visa-resource-name>, error out=w397:errorcluster)  [unwired: 1 out]
        n203 = property class="Instr"(reference=w396, error in=w397) -> (reference out=w395:refnum<visa-resource-name>, error out=w394:errorcluster, "Serial Settings:Number of Bytes at Serial Port"=w393:u32)
        n204 = VISA Read(VISA resource name=w395, byte count=w393, error in (no error)=w394) -> (VISA resource name out=w401:refnum<visa-resource-name>, error out=w400:errorcluster)  [unwired: 2 out]
      }
      event "停止运动": Mouse Down {
        n205 = event-data() -> ()  [unwired: 1 in, 8 out]
        n206 = Concatenate Strings("I" ("写入缓冲区"), "\r") -> (w406:string)
        n207 = VISA Write ("VISA写入")(VISA resource name=w405, write buffer=w406, error in (no error)=w404) -> (VISA resource name out=w412:refnum<visa-resource-name>, error out=w413:errorcluster)  [unwired: 1 out]
        n208 = property class="Instr"(reference=w412, error in=w413) -> (reference out=w411:refnum<visa-resource-name>, error out=w410:errorcluster, "Serial Settings:Number of Bytes at Serial Port"=w409:u32)
        n209 = VISA Read(VISA resource name=w411, byte count=w409, error in (no error)=w410) -> (VISA resource name out=w403:refnum<visa-resource-name>, error out=w402:errorcluster)  [unwired: 2 out]
      }
      event "设置移动步长": Mouse Down; "调焦步伐/um": Value Change {
        n210 = event-data() -> ()  [unwired: 1 in, 4 out]
        n211 = Add(x="调焦步伐/um", y=i64 1) -> (x+y=w414:i64)
        n212 = Power Of 10(x=w414) -> (10^x=w417:dbl)
        n213 = Number To Decimal String(number=w417) -> (decimal integer string=w418:string)  [unwired: 1 in]
        n214 = Concatenate Strings("C," ("写入缓冲区"), w418, "\r") -> (w424:string)
        n215 = VISA Write ("VISA写入")(VISA resource name=w423, write buffer=w424, error in (no error)=w422) -> (VISA resource name out=w429:refnum<visa-resource-name>, error out=w430:errorcluster)  [unwired: 1 out]
        n216 = property class="Instr"(reference=w429, error in=w430) -> (reference out=w428:refnum<visa-resource-name>, error out=w427:errorcluster, "Serial Settings:Number of Bytes at Serial Port"=w426:u32)
        n217 = VISA Read(VISA resource name=w428, byte count=w426, error in (no error)=w427) -> (VISA resource name out=w421:refnum<visa-resource-name>, error out=w420:errorcluster)  [unwired: 2 out]
      }
      event "返回Z轴坐标": Mouse Down {
        n218 = event-data() -> ()  [unwired: 1 in, 8 out]
        n219 = Concatenate Strings("PZ" ("写入缓冲区"), "\r") -> (w441:string)
        n220 = VISA Write ("VISA写入")(VISA resource name=w439, write buffer=w441, error in (no error)=w438) -> (VISA resource name out=w435:refnum<visa-resource-name>, error out=w434:errorcluster)  [unwired: 1 out]
        n221 = flat-sequence {
          tunnel: w435 -> [w447]
          tunnel: w434 -> [w448]
          tunnel: [w448] -> w432
          tunnel: [w447] -> w433
          frame #0 {
            # "发送命令需要等一下"
            n222 = Wait (ms)(milliseconds to wait=u32 30 ("等待时间（毫秒）")) -> ()  [unwired: 1 out]
          }
        }
        n223 = property class="Instr"(reference=w433, error in=w432) -> (reference out=w445:refnum<visa-resource-name>, error out=w444:errorcluster, "Serial Settings:Number of Bytes at Serial Port"=w443:u32)
        n224 = VISA Read(VISA resource name=w445, byte count=w443, error in (no error)=w444) -> (VISA resource name out=w437:refnum<visa-resource-name>, read buffer=→"读取缓冲区":string, error out=w436:errorcluster)  [unwired: 1 out]
      }
      event "up": Mouse Down {
        n225 = event-data() -> ()  [unwired: 1 in, 8 out]
        n226 = Concatenate Strings("U" ("写入缓冲区"), "\r") -> (w454:string)
        n227 = VISA Write ("VISA写入")(VISA resource name=w458, write buffer=w454, error in (no error)=w457) -> (VISA resource name out=w453:refnum<visa-resource-name>, error out=w452:errorcluster)  [unwired: 1 out]
        n228 = property class="Instr"(reference=w453, error in=w452) -> (reference out=w450:refnum<visa-resource-name>, error out=w449:errorcluster, "Serial Settings:Number of Bytes at Serial Port"=w451:u32)
        n229 = VISA Read(VISA resource name=w450, byte count=w451, error in (no error)=w449) -> (VISA resource name out=w460:refnum<visa-resource-name>, error out=w459:errorcluster)  [unwired: 2 out]
      }
    }
    n230 = Unbundle By Name(w368) -> ("status"=w364:bool)
  }
  n231 = while {
    tunnel: w108 -> [w470]
    tunnel: [w469] -> w39
    tunnel: w2 -> [w468]
    tunnel: w1 -> [w467]
    stop <- w465 stop-if-true
    # "电流信号循环"
    n232 = Dequeue Element(queue=w468, timeout in ms (-1)=1 ("超时毫秒(-1)"), error in (no error)=w467) -> (error out=w463:errorcluster)  [unwired: 3 out]
    n233 = flat-sequence {
      tunnel: w470 -> [w491]
      tunnel: [w491] -> w462
      tunnel: [w479] -> w461
      tunnel: [w499] -> w472
      tunnel: [w514] -> w471
      tunnel: w462 -> [w500]
      tunnel: w461 -> [w514]
      tunnel: [w535] -> w476
      tunnel: [w520] -> w475
      tunnel: w472 -> [w515]
      tunnel: w471 -> [w531]
      tunnel: w476 -> [w610]
      tunnel: w475 -> [w611]
      tunnel: w470 -> [w612]
      tunnel: [w609] -> w474
      tunnel: [w601] -> w473
      tunnel: [w654] -> w469
      tunnel: w474 -> [w654]
      tunnel: w473 -> [w652]
      frame #0 {
        n234 = case shown="真" "控制箱刺激ON\n/放大器刺激" {
          tunnel: [0.0 ("data") 5.0 ("data")] -> w488
          frame False {
          }
          frame True {
          }
        }
        n235 = call-poly <vilib>:"DAQmx Create Virtual Channel.vi"("physical channels"=tag "Dev2/ao1") -> ("task out"=w484:refnum<k21>, "error out"=w485:errorcluster)  [unwired: 13 in]
        n236 = call <vilib>:"DAQmx Start Task.vi"("task/channels in"=w484, "error in"=w485) -> ("task out"=w483:refnum<k21>, "error out"=w482:errorcluster)  [unwired: 12 in]
        n237 = call-poly <vilib>:"DAQmx Write.vi"("task/channels in"=w483, "data"=w488, "error in"=w482) -> ("task out"=w481:refnum<k21>, "error out"=w480:errorcluster)  [unwired: 10 in, 1 out]
        n238 = call <vilib>:"DAQmx Stop Task.vi"("task/channels in"=w481, "error in"=w480) -> ("task out"=w487:refnum<k21>, "error out"=w486:errorcluster)  [unwired: 12 in]
        n239 = call <vilib>:"DAQmx Clear Task.vi"("task in"=w487, "error in"=w486) -> ("error out"=w479:errorcluster)  [unwired: 13 in]
      }
      frame #1 {
        n240 = Unbundle By Name(w500) -> ("amplitude"=w506:dbl, "frequency"=w505:dbl, "Fs"=w507:dbl, "Averaging"=w508:i32)
        n241 = Multiply(x=w507, y=w508) -> (x*y=w503:dbl)
        n242 = Multiply(x="钳制电位", y="Holding Voltage") -> (x*y=w496:dbl)
        n243 = Divide(x=w503, y=w505) -> (x/y=w504:dbl)
        n244 = Divide(x=w506, y=2.0) -> (x/y=w510:dbl)
        n245 = Add(x=w496, y=0.5) -> (x+y=w494:dbl)
        "x*y" <- w494
        n246 = Divide(x=w494, y=1000.0) -> (x/y=w511:dbl)
        n247 = Add(x=w511, y=w510) -> (x+y=w501:dbl)
        n248 = Bundle("Fs"=w507, w504) -> (w509:cluster{"Fs":dbl, dbl})  [unwired: 1 in]
        n249 = call <vilib>:"Basic Function Generator.vi"("offset"=w501, "sampling info"=w509, "signal type"=T10."Square Wave", "amplitude"=w510, "frequency"=w505) -> ("signal out"=w499:waveform(dbl))  [unwired: 4 in, 2 out]
      }
      frame #2 {
        w564 = 10178 items=["有限采样"=10178, "连续采样"=10123, "硬件定时单点"=12522] ("sample mode")
        w565 = tag "OnboardClock" ("source")
        w557 = 10178 items=["有限采样"=10178, "连续采样"=10123, "硬件定时单点"=12522] ("sample mode")
        # "必须要有触发"
        # "This version of StimRecord is for the NI DAQ used in conjunction with the MultiClamp 700b"
        # "multiclamp放大器自己参数"
        # "in V"
        # "in nA"
        n250 = case shown="1" "下拉列表" {
          tunnel: [50.0 ("y") 2500000000.0 ("y")] -> w532
          tunnel: [2000.0 ("y") 0.1 ("y")] -> w533
          frame 0, Default {
          }
          frame 1 {
          }
        }
        n251 = Multiply(x=w515, y=w532) -> (x*y=w550:waveform(dbl))
        n252 = call-poly <vilib>:"Waveform Duration.vi"("waveform in"=w515) -> ("duration"=w552:dbl)  [unwired: 8 in, 2 out]
        n253 = Unbundle By Name(w550) -> ("Y"=w519:dbl[], "dt"=w549:dbl)
        n254 = for {
          tunnel: [w579] -> w518 mode=indexing
          tunnel: w519 -> [w573] mode=indexing
          w574 = 10.0 ("t")
          w577 = -10.0 ("t")
          n255 = Greater?(x=w577, y=w573) -> (0:w578:bool)
          n256 = Select(t=w577, s=w578, f=w573) -> (s? t:f=w575:dbl)
          n257 = Less?(x=w574, y=w575) -> (x < y?=w576:bool)
          n258 = Select(t=w574, s=w576, f=w575) -> (s? t:f=w579:dbl)
        }
        n259 = Multiply(x=w552, y=2.0) -> (x*y=w553:dbl)
        n260 = Add(x=w553, y=5.0) -> (x+y=w522:dbl)
        n261 = call-poly <vilib>:"DAQmx Create Virtual Channel.vi"("physical channels"=tag "Dev2/ai0", "error in"=w531) -> ("task out"=w556:refnum<k21>, "error out"=w555:errorcluster)  [unwired: 12 in]
        n262 = call-poly <vilib>:"DAQmx Create Virtual Channel.vi"("physical channels"=tag "Dev2/ao0", "error in"=w531) -> ("task out"=w545:refnum<k21>, "error out"=w544:errorcluster)  [unwired: 12 in]
        n263 = Reciprocal(x=w549) -> (1/x=w558:dbl)
        n264 = Array Size(array=w519) -> (size(s)=w572:i32)
        n265 = call-poly <vilib>:"DAQmx Timing.vi"("task/channels in"=w545, "sample mode"=w564, "samples per channel"=w572, "rate"=w558, "source"=w565, "error in"=w544) -> ("task out"=w530:refnum<k21>, "error out"=w528:errorcluster)  [unwired: 8 in]
        n266 = Bundle By Name(cluster=w550, "Y"=w518) -> (w551:waveform(dbl))
        n267 = call-poly <vilib>:"DAQmx Timing.vi"("task/channels in"=w556, "sample mode"=w557, "samples per channel"=w572, "rate"=w558, "source"=w565, "error in"=w555) -> ("task out"=w560:refnum<k21>, "error out"=w561:errorcluster)  [unwired: 8 in]
        n268 = call-poly <vilib>:"DAQmx Trigger.vi"("task/channels in"=w530, "source"=tag "/Dev2/ai/StartTrigger", "error in"=w528) -> ("task out"=w529:refnum<k21>, "error out"=w527:errorcluster)  [unwired: 11 in]
        n269 = call-poly <vilib>:"DAQmx Write.vi"("task/channels in"=w529, "auto start"=FALSE, "data"=w551, "timeout"=w522, "error in"=w527) -> ("task out"=w548:refnum<k21>, "error out"=w569:errorcluster)  [unwired: 8 in, 1 out]
        n270 = property class="DAQmx定时" props=["SampClk.Rate"](reference=w560, error in=w561) -> (reference out=w562:refnum<k21>)  [unwired: 2 out]
        n271 = call <vilib>:"DAQmx Start Task.vi"("task/channels in"=w548, "error in"=w569) -> ("task out"=w566:refnum<k21>, "error out"=w568:errorcluster)  [unwired: 12 in]
        n272 = call <vilib>:"DAQmx Start Task.vi"("task/channels in"=w562, "error in"=w568) -> ("task out"=w540:refnum<k21>, "error out"=w541:errorcluster)  [unwired: 12 in]
        n273 = call-poly <vilib>:"DAQmx Read.vi"("task/channels in"=w540, "number of samples per channel"=w572, "timeout"=w522, "error in"=w541) -> ("task out"=w526:refnum<k21>, "data"=w554:waveform(dbl), "error out"=w524:errorcluster)  [unwired: 9 in]
        n274 = call <vilib>:"DAQmx Is Task Done.vi"("task/channels in"=w566, "error in"=w568) -> ("task out"=w567:refnum<k21>, "error out"=w570:errorcluster)  [unwired: 11 in, 1 out]
        n275 = call <vilib>:"DAQmx Wait Until Done.vi"("task/channels in"=w567, "timeout (sec)"=w522, "error in"=w570) -> ("task out"=w546:refnum<k21>, "error out"=w547:errorcluster)  [unwired: 11 in]
        n276 = call <vilib>:"DAQmx Wait Until Done.vi"("task/channels in"=w526, "timeout (sec)"=w522, "error in"=w524) -> ("task out"=w525:refnum<k21>, "error out"=w523:errorcluster)  [unwired: 11 in]
        n277 = call <vilib>:"DAQmx Stop Task.vi"("task/channels in"=w546, "error in"=w547) -> ("task out"=w543:refnum<k21>, "error out"=w542:errorcluster)  [unwired: 12 in]
        n278 = Multiply(x=w554, y=w533) -> (x*y=w520:waveform(dbl))
        "电流信号波形图" <- w520
        n279 = call <vilib>:"DAQmx Stop Task.vi"("task/channels in"=w525, "error in"=w523) -> ("task out"=w538:refnum<k21>, "error out"=w539:errorcluster)  [unwired: 12 in]
        n280 = call <vilib>:"DAQmx Clear Task.vi"("task in"=w543, "error in"=w542) -> ("error out"=w571:errorcluster)  [unwired: 13 in]
        n281 = call <vilib>:"DAQmx Clear Task.vi"("task in"=w538, "error in"=w539) -> ("error out"=w537:errorcluster)  [unwired: 13 in]
        n282 = Merge Errors(w571, w537) -> (w535:errorcluster)
        n283 = Build Array(w550, w520) -> ()  [unwired: 1 out]
      }
      frame #3 {
        # "数据读取错误"
        # "阻值读取异常处理"
        # "单位换算不明白"
        # "阻值处理"
        # "Convert Volts/pA into MOhms"
        n284 = call "Filter"("error in (no error)"=w610, "Signal"=w611) -> ("error out"=w613:errorcluster, "Filtered Signal"=w605:dynamicdata)  [unwired: 8 in]
        n285 = call "单频测量"("Signals"=w605) -> ("Frequency"=w604:dynamicdata)  [unwired: 9 in, 1 out]
        n286 = Unbundle By Name(w612) -> ("Fs"=w626:dbl, "frequency"=w625:dbl, "Proportion"=w618:dbl)
        n287 = Unbundle By Name(w612) -> ("Averaging"=w624:i32)
        n288 = call "Convert from Dynamic Data"("Dynamic Data Type"=w605) -> ("Array"=w616:dbl[])  [unwired: 3 in]
        n289 = call "从动态数据转换"("Dynamic Data Type"=w604) -> ("Array"=w603:dbl[])  [unwired: 3 in]
        n290 = call-poly <vilib>:"Mean.vi"("X"=w603) -> ("mean"=w600:dbl)  [unwired: 1 out]
        n291 = Divide(x=w626, y=w625) -> (x/y=w629:dbl)
        n292 = Reshape Array(w616, w624, w629) -> (w628:dbl[][])
        n293 = call-poly <vilib>:"Mean.vi"("X"=w616) -> ("mean"=w617:dbl)  [unwired: 1 out]
        n294 = for {
          N: w624 -> [_]
          tunnel: w628 -> [w640] mode=indexing
          tunnel: w613 -> [w647]
          shift-right: [w648] -> w627
          shift-left: dbl[] [] -> [w649]
          tunnel: [w635] -> w623
          tunnel: [w647] -> w609
          tunnel: w618 -> [w639]
          # "不是整个电流的均值"
          # "波形后半段"
          # "波形前半段"
          n295 = Array Size(array=w640) -> (size(s)=w637:i32)
          n296 = Subtract(x=1.0, y=w639) -> (x-y=w642:dbl)
          n297 = Divide(x=w637, y=2) -> (x/y=w644:dbl)
          n298 = Multiply(x=w644, y=w642) -> (x*y=w641:dbl)
          n299 = Split 1D Array(array=w640, index=w644) -> (first subarray=w636:dbl[], second subarray=w645:dbl[])
          n300 = Split 1D Array(array=w636, index=w641) -> (second subarray=w632:dbl[])  [unwired: 1 out]
          n301 = Split 1D Array(array=w645, index=w641) -> (second subarray=w633:dbl[])  [unwired: 1 out]
          n302 = call-poly <vilib>:"Mean.vi"("X"=w632) -> ("mean"=w634:dbl)  [unwired: 1 out]
          n303 = call-poly <vilib>:"Mean.vi"("X"=w633) -> ("mean"=w635:dbl)  [unwired: 1 out]
          n304 = Subtract(x=w634, y=w635) -> (x-y=w638:dbl)
          n305 = Build Array (concatenate)(w649, w638) -> (w648:dbl[])
        }
        "Negative Peak" <- w623
        n306 = Subtract(x=w600, y=sgl 20.0) -> (x-y=w598:dbl)
        n307 = Array Max & Min(array=w616) -> (min value=w615:dbl)  [unwired: 3 out]
        n308 = Absolute Value(x=w598) -> (abs(x)=w597:dbl)
        n309 = Greater?(x=w597, y=0.05) -> (0:w591:bool)
        "！" <- w591
        n310 = Subtract(x=w617, y=w615) -> (x-y=w614:dbl)
        n311 = Unbundle By Name(w612) -> ("amplitude"=w621:dbl)
        n312 = Multiply(x=w621, y=1000000.0) -> (x*y=w608:dbl)
        n313 = Divide(x=w608, y=w614) -> (x/y=→"电阻值":dbl)
        n314 = call-poly <vilib>:"Mean.vi"("X"=w627) -> ("mean"=w622:dbl)  [unwired: 1 out]
        n315 = local read "Resistance(MΩ)"() -> (w594:dbl)
        n316 = Divide(x=w608, y=w622) -> (x/y=w607:dbl)
        n317 = Multiply(x=w607, y=2.0) -> (x*y=w606:dbl)
        n318 = local read "阻值数组"() -> (w602:dbl[])
        n319 = Less?(x=w594, y=100.0) -> (x < y?=w592:bool)
        n320 = And(x=w592, y=w591) -> (x .and. y?=w590:bool)
        n321 = case shown="假" w590 {
          tunnel: w594 -> [_ w631]
          tunnel: w606 -> [w630 _]
          tunnel: [w630 w631] -> w589
          frame False {
          }
          frame True {
          }
        }
        n322 = In Range and Coerce(upper limit=10000.0 ("上限"), x=w589, lower limit=0.0 ("下限")) -> (coerced(x)=w584:dbl)  [unwired: 1 out]
        "阻值波形图表" <- w584
        "Resistance(MΩ)" <- w584
        n323 = Insert Into Array(array=w602, index=0 ("索引"), new element=w584) -> (w601:dbl[])
        n324 = local write "阻值数组"(w601) -> ()
      }
      frame #4 {
        n325 = Array Size(array=w652) -> (size(s)=w651:i32)
        n326 = Greater?(x=w651, y=10) -> (0:w650:bool)
        n327 = case shown="真" w650 {
          tunnel: w652 -> [_ w658]
          frame False {
          }
          frame True {
            n328 = Delete From Array(array=w658, length=1 ("长度"), index=9 ("索引")) -> (array with subset deleted=w655:dbl[])  [unwired: 1 out]
            n329 = local write "阻值数组"(w655) -> ()
          }
        }
      }
    }
    n330 = Unbundle By Name(w463) -> ("status"=w465:bool)
    n331 = case shown="真" "入液阻值校准" {
      frame False {
      }
      frame True {
        n332 = flat-sequence {
          frame #0 {
            n333 = local read "Resistance(MΩ)"() -> (→"校准的入液阻值":dbl)
          }
          frame #1 {
            n334 = local write "入液阻值校准"(FALSE) -> ()
          }
        }
      }
    }
  }
  n335 = VISA Close(VISA resource name=w4, error in (no error)=w3) -> ()  [unwired: 1 out]
  n336 = call "IMAQ Create"("Image Name"="二值化") -> ("New Image"=w42:T1)  [unwired: 4 in, 1 out]
  n337 = call "IMAQ Create"("Image Name"="针尖清晰度图像处理") -> ("New Image"=w43:T1)  [unwired: 4 in, 1 out]
  n338 = call "IMAQ Create"("Image Name"="图像检测") -> ("New Image"=w11:T1)  [unwired: 4 in, 1 out]
  n339 = call "IMAQ Create"("Image Name"="mask图像") -> ("New Image"=w9:T1)  [unwired: 4 in, 1 out]
  n340 = while {
    tunnel: w118 -> [w695]
    tunnel: w116 -> [w694]
    tunnel: [w693] -> w111
    shift-right: [w691] -> _
    shift-left: _ -> [w690]
    tunnel: w109 -> [w688]
    tunnel: [w671] -> w107
    tunnel: [w687] -> w106
    tunnel: w105 -> [w686]
    tunnel: [w685] -> w104
    tunnel: w103 -> [w684]
    tunnel: w2 -> [w683]
    tunnel: [w680] -> w101
    shift-right: [w679] -> w100
    shift-left: w1 -> [w678]
    tunnel: w46 -> [w672]
    tunnel: w43 -> [w670]
    tunnel: w42 -> [w669]
    tunnel: w11 -> [w661]
    tunnel: w9 -> [w660]
    stop <- "停止" stop-if-true
    (unwired) 2 ("长度")
    # "图像检测"
    # "图像处理循环"
    # "目标坐标"
    n341 = property on="Image" class="ImageControl"() -> ("ROI"=w674:T11)  [unwired: 2 in, 2 out]
    n342 = Unbundle(w674) -> ("Global Rectangle"=w676:i32[])  [unwired: 1 out]
    n343 = Tick Count (ms)() -> (millisecond timer value=w691:u32)
    n344 = call <vilib>:"IMAQdx Grab2.vi"("error in"=w686, "Image In"=w694, "Session In"=w695) -> ("error out"=w685:errorcluster, "Image Out"=w689:T1, "Session Out"=w693:T6)  [unwired: 5 in, 1 out]
    n345 = Array Subset(array=w676, index=0 ("索引")) -> (→"目标坐标":i32[])  [unwired: 1 in]
    n346 = Subtract(x=w691, y=w690) -> (x-y=→"循环时间":u32)
    n347 = call "IMAQ ExtractSingleColorPlane"("error in (no error)"=w684, "Image Dst"=w688, "Image Src"=w689) -> ("error out"=w687:errorcluster, "Image Dst Out"=w671:T1)  [unwired: 7 in]
    n348 = Enqueue Element(queue=w683, element="停止", timeout in ms (-1)=1 ("超时毫秒(-1)"), error in (no error)=w678) -> (queue out=w680:refnum<queue>, error out=w679:errorcluster)  [unwired: 1 out]
    n349 = case shown="真" "针尖模板匹配" {
      tunnel: w672 -> [_ w796]
      tunnel: w671 -> [w756 w760]
      tunnel: [FALSE w795] -> w665
      tunnel: [w755 w763] -> _
      tunnel: [w756 w759] -> w663
      frame False {
        w757 = 0.0 ("x")
        n350 = Bundle("x"=w757, "x"=w757) -> (w755:cluster{"x":dbl, "x":dbl})  [unwired: 1 in]
      }
      frame True {
        w762 = u32 1 items=["Frame", "Fill", "Highlight"] ("Drawing Mode (Frame)")
        w765 = 10.0 ("y")
        w789 = u16 0 items=["All", "Shift Information", "Rotation Information"] ("Learn Mode")
        # "目标和针尖坐标获取"
        # "模板针尖偏移量"
        # "是否匹配到"
        # "模板匹配针尖"
        n351 = call "IMAQ Setup Match Pattern 2"("Minimum Contrast"="Minimum Contrast", "Match Mode"="Match Mode") -> ("Match Pattern Setup Data"=w793:string)  [unwired: 8 in, 1 out]
        n352 = call "IMAQ Setup Learn Pattern 2"("Learn Mode"=w789) -> ("Learn Pattern Setup Data"=w788:string)  [unwired: 9 in, 1 out]
        n353 = call "IMAQ Learn Pattern 2"("Learn Pattern Setup Data"=w788, "Image"=w796) -> ("Template Image Out"=w785:T1)  [unwired: 8 in, 1 out]
        n354 = call "IMAQ Match Pattern 2"("Minimum Match Score"="Minimum Match Score", "Number of Matches Requested"="Number of Matches Requested", "Match Pattern Setup Data"=w793, "Template Image"=w785, "Image"=w760) -> ("Number of Matches"=w786:i32, "Matches"=w782:T5)  [unwired: 4 in, 1 out]
        "Number of Matches" <- w786
        "Matches 2" <- w782
        n355 = Equal?(x=w786, y=0) -> ()  [unwired: 1 out]
        n356 = Index Array(array=w782, index=0 ("索引")) -> (element=w780:T12)
        n357 = Index Array(array=w782, index=0 ("索引")) -> (element=w764:T12)
        n358 = Unbundle(w780) -> ("Score"=w779:sgl)  [unwired: 4 out]
        n359 = Less?(x=w779, y=sgl 800.0) -> (x < y?=w795:bool)
        n360 = Unbundle(w764) -> ("Position"=w763:cluster{"x":sgl, "y":sgl})  [unwired: 4 out]
        n361 = Cluster To Array(cluster=w763) -> (array=→"针尖坐标":sgl[])
        n362 = Unbundle(w763) -> ("x"=w774:sgl, "y"=w777:sgl)
        n363 = Add(x=w774, y=sgl 0.0) -> (x+y=w776:sgl)
        n364 = Subtract(x=w777, y=w765) -> (x-y=w768:dbl)
        n365 = Add(x=w777, y=w765) -> (x+y=w767:dbl)
        n366 = Subtract(x=w776, y=w765) -> (x-y=w766:dbl)
        n367 = Add(x=w776, y=w765) -> (x+y=w769:dbl)
        n368 = To Long Integer(number=w768) -> (32bit integer=w771:i32)
        n369 = To Long Integer(number=w767) -> (32bit integer=w772:i32)
        n370 = To Long Integer(number=w766) -> (32bit integer=w770:i32)
        n371 = To Long Integer(number=w769) -> (32bit integer=w773:i32)
        n372 = Bundle(w770, w771, w773, w772) -> (w761:cluster{i32, i32, i32, i32})  [unwired: 1 in]
        n373 = call "IMAQ Overlay Oval"("Drawing Mode (Frame)"=w762, "Bounding Rectangle"=w761, "Image"=w760) -> ("Image Out"=w759:T1)  [unwired: 7 in, 1 out]
      }
    }
    "Image" <- w663
    "是否匹配到？" <- w665
    n374 = case shown="真" "对比图" {
      tunnel: w663 -> [_ w720]
      frame False {
      }
      frame True {
        n375 = flat-sequence {
          tunnel: w720 -> [w721]
          frame #0 {
            "Image 2" <- w721
          }
          frame #1 {
            n376 = local write "对比图"(FALSE) -> ()
          }
        }
      }
    }
    n377 = local read "针尖细对焦"() -> (w666:bool)
    n378 = local read "针尖粗对焦"() -> (w667:bool)
    n379 = Or(x=w667, y=w666) -> (x .or. y?=w659:bool)
    n380 = case shown="真" w659 {
      tunnel: [0.0 ("Right") w739] -> w668
      tunnel: w663 -> [_ w726]
      tunnel: w670 -> [_ w725]
      tunnel: w669 -> [_ w724]
      frame False {
      }
      frame True {
        n381 = call "IMAQ Threshold"("Range"="Range", "Image Dst"=w724, "Image Src"=w726) -> ("Image Dst Out"=w729:T1)  [unwired: 7 in, 1 out]
        n382 = call "IMAQ LowPass"("Image Src"=w729) -> ("Image Dst Out"=w730:T1)  [unwired: 6 in, 1 out]
        n383 = call "IMAQ Copy"("Image Dst"=w725, "Image Src"=w730) -> ("Image Dst Out"=w737:T1)  [unwired: 4 in, 1 out]
        n384 = call "IMAQ RemoveParticle"("Number of Erosion"="Number of Erosion", "Image Src"=w737) -> ("Image Dst Out"=w731:T1)  [unwired: 8 in, 1 out]
        n385 = call "IMAQ Morphology"("Operation"="Operation", "Image Src"=w731) -> ("Image Dst Out"=w734:T1)  [unwired: 8 in, 1 out]
        n386 = call "IMAQ Convex Hull"("Image Src"=w734) -> ("Image Dst Out"=w735:T1)  [unwired: 9 in, 1 out]
        n387 = call "IMAQ FillHole"("Image Src"=w735) -> ("Image Dst Out"=w732:T1)  [unwired: 5 in, 1 out]
        n388 = call "IMAQ Clear Overlay"("Image"=w732) -> ("Image Out"=w728:T1)  [unwired: 9 in, 1 out]
        "二值化" <- w728
        n389 = call "IMAQ Particle Analysis Report"("Image"=w728) -> ("Particle Reports (Pixels)"=w727:T4)  [unwired: 5 in, 5 out]
        "Particle Reports (Pixels)" <- w727
        n390 = while {
          tunnel: w727 -> [w740]
          shift-right: [w749] -> w739
          shift-left: _ -> [w744]
          i -> [w742]
          stop <- w746 stop-if-true
          n391 = Equal?(x=w742, y=0) -> (x = y?=w743:bool)
          n392 = case shown="假" w743 {
            tunnel: w744 -> [w753 _]
            tunnel: [w753 0] -> w741
            frame False {
            }
            frame True {
            }
          }
          n393 = Index Array(array=w740, index=w742) -> (element=w751:T13)
          n394 = Unbundle(w751) -> ("Bounding Rect"=w752:T14)  [unwired: 5 out]
          n395 = Unbundle(w752) -> ("Right"=w747:dbl)  [unwired: 3 out]
          n396 = Equal?(x=w747, y=0.0) -> (x = y?=w746:bool)
          n397 = Greater?(x=w741, y=w747) -> (0:w750:bool)
          n398 = Select(t=w741, s=w750, f=w747) -> (s? t:f=w749:dbl)
        }
        "Right" <- w739
      }
    }
    "清晰度评价函数" <- w668
    n399 = local read "自动接触"() -> (w662:bool)
    n400 = case shown="真" w662 {
      tunnel: w661 -> [_ w717]
      tunnel: w660 -> [_ w700]
      frame False {
      }
      frame True {
        w699 = 200 ("image_size")
        n401 = local read "目标坐标"() -> (w709:i32[])
        n402 = local read "针尖坐标"() -> (w712:sgl[])
        n403 = local read "Image 2"() -> (w718:T1)
        n404 = local read "Image"() -> (w719:T1)
        n405 = Index Array(array=w712, index=1 ("索引")) -> (element=w703:sgl)
        n406 = Index Array(array=w712, index=0 ("索引")) -> (element=w704:sgl)
        n407 = Index Array(array=w709, index=1 ("索引")) -> (element=w705:i32)
        n408 = Index Array(array=w709, index=0 ("索引")) -> (element=w706:i32)
        n409 = call "IMAQ Absolute Difference"("Image Src A"=w719, "Image Dst"=w717, "Image Src B"=w718) -> ("Image Dst Out"=w714:T1)  [unwired: 4 in, 1 out]
        n410 = call "IMAQ ImageToArray"("Image"=w714) -> ("Image Pixels (U8)"=w713:u8[][])  [unwired: 3 in, 4 out]
        n411 = call "IMAQ GetImageSize"("Image"=w714) -> ("Y Resolution"=w715:i32, "X Resolution"=w716:i32)  [unwired: 3 in, 1 out]
        n412 = Initialize Array(u8 0 ("元素"), w699, w699) -> (w697:u8[][])
        n413 = dll-call lib="PTH2=abs E膜片\t膜片钳程序vscellDebugcell.dll" fn="DeformationDetect"("rows"=w715, "cols"=w716, "image"=w713, "cell_X"=w706, "cell_Y"=w705, "tip_X"=w704, "tip_Y"=w703, "data"=w697, "image_size"=w699) -> ("cout"=→"cout":i32, "data"=w696:u8[][])  [unwired: 11 in, 2 out]
        n414 = call "IMAQ ArrayToImage"("Image Pixels (U8)"=w696, "Image"=w700) -> ("Image Out"=→"Image 3":T1)  [unwired: 8 in, 1 out]
      }
    }
  }
  n415 = Get Date/Time String(date format (0)=enum16{"short", "long", "abbreviated"}."long" ("日期格式(0)"), want seconds? (F)=TRUE ("需要秒？(F)")) -> (date string=w35:string, time string=w20:string)  [unwired: 1 in]
  n416 = String Subset(string=w20, offset (0)=6 ("偏移量(0)")) -> (substring=w18:string)  [unwired: 1 in]
  n417 = String Subset(string=w20, offset (0)=3 ("偏移量(0)"), length (rest)=2 ("长度（剩余）")) -> (substring=w30:string)
  n418 = String Subset(string=w20, length (rest)=2 ("长度（剩余）")) -> (substring=w32:string)  [unwired: 1 in]
  n419 = Concatenate Strings(w32, "时" ("字符串"), w30, "分" ("字符串"), w18, "秒" ("字符串")) -> (w31:string)
  n420 = Concatenate Strings(w35, w31) -> (w14:string)
  n421 = call "SetDA.vi"("错误输入（无错误）"=w7, "DevIndex"=w8) -> ("错误输出"=w72:errorcluster, "DevIndex Output"=w73:i32)  [unwired: 8 in]
  n422 = Build Path(base path=path "E:/膜片/实验/数据" ("文件路径（使用对话框）"), name or relative path=w14) -> (appended path=w28:path)
  n423 = call "SetDA.vi"("错误输入（无错误）"=w72, "DAVolt"=0.0, "DANum"=u8 1, "DevIndex"=w73) -> ("错误输出"=w71:errorcluster, "DevIndex Output"=w70:i32)  [unwired: 6 in]
  n424 = Create Folder(path (use dialog)=w28) -> (created path=w23:path)  [unwired: 2 in, 2 out]
  n425 = Build Path(base path=w23, name or relative path="data.txt" ("字符串")) -> (appended path=w25:path)
  n426 = Build Array(w61, w61, w61, w61, w61, w61, w61, w61) -> (w59:bool[])
  n427 = call "SetDA.vi"("错误输入（无错误）"=w71, "DAVolt"=0.0, "DANum"=u8 2, "DevIndex"=w70) -> ("错误输出"=w68:errorcluster, "DevIndex Output"=w69:i32)  [unwired: 6 in]
  n428 = Open/Create/Replace File(file path (use dialog)=w25, operation (0:open)=T7."open or create" ("操作(0:open)")) -> (refnum out=w24:refnum<file>)  [unwired: 4 in, 2 out]
  n429 = while {
    tunnel: w41 -> [w810]
    tunnel: w1 -> [w813]
    tunnel: [w803] -> w37
    tunnel: w2 -> [w812]
    tunnel: w24 -> [w801]
    tunnel: w23 -> [w800]
    tunnel: [w798] -> w22
    i -> [w799]
    stop <- w814 stop-if-true
    # "Mp285A控制循环"
    n430 = Dequeue Element(queue=w812, timeout in ms (-1)=1 ("超时毫秒(-1)"), error in (no error)=w813) -> (error out=w815:errorcluster)  [unwired: 3 out]
    n431 = Unbundle By Name(w815) -> ("status"=w814:bool)
    n432 = flat-sequence {
      tunnel: [w901] -> w811
      tunnel: w810 -> [w901]
      tunnel: w811 -> [w908]
      tunnel: [w907] -> w809
      tunnel: w809 -> [w987]
      tunnel: [w986] -> w808
      frame #0 {
        n433 = event shown="[1] 超时" {
          selector: _ -> [_ _]
          dyn-events: _ -> [_ _]
          timeout: 1 -> [_ _]
          event "针尖粗对焦": Mouse Down {
            n434 = event-data() -> ()  [unwired: 1 in, 8 out]
            n435 = Array Size(array="聚焦值数组") -> (size(s)=w903:i32)
            n436 = Delete From Array(array="聚焦值数组", length=w903) -> (array with subset deleted=w904:dbl[])  [unwired: 1 in, 1 out]
            n437 = local write "聚焦值数组"(w904) -> ()
            "布尔" <- TRUE
          }
          event Timeout {
            n438 = event-data() -> ()  [unwired: 1 in, 3 out]
          }
        }
      }
      frame #1 {
        n439 = local read "Right"() -> (w909:dbl)
        n440 = case shown="真" "针尖粗对焦" {
          tunnel: w909 -> [_ w916]
          tunnel: w908 -> [w912 w914]
          tunnel: [w912 w913] -> w907
          frame False {
            n441 = local write "布尔"(FALSE) -> ()
          }
          frame True {
            # "爬山算法"
            # "聚焦有问题"
            n442 = flat-sequence {
              tunnel: w916 -> [w974]
              tunnel: [w984] -> w921
              tunnel: [w983] -> w919
              tunnel: [w982] -> w920
              frame #0 {
                n443 = local read "布尔"() -> (w973:bool)
                n444 = case shown="假" w973 {
                  tunnel: w974 -> [w975 w979]
                  frame False {
                    n445 = flat-sequence {
                      tunnel: w975 -> [w978]
                      frame #0 {
                        n446 = local read "调焦值 3"() -> (w976:dbl)
                        n447 = local write "调焦值 4"(w976) -> ()
                      }
                      frame #1 {
                        n448 = local read "调焦值2"() -> (w977:dbl)
                        n449 = local write "调焦值 3"(w977) -> ()
                      }
                      frame #2 {
                        n450 = local write "调焦值2"(w978) -> ()
                      }
                    }
                  }
                  frame True {
                    # "第一次赋值"
                    "调焦值2" <- w979
                    "调焦值 3" <- w979
                    "调焦值 4" <- w979
                    "变量" <- 1
                  }
                }
              }
              frame #1 {
                n451 = local write "布尔"(FALSE) -> ()
              }
              frame #2 {
                n452 = local read "调焦值2"() -> (w984:dbl)
                n453 = local read "调焦值 3"() -> (w983:dbl)
                n454 = local read "调焦值 4"() -> (w982:dbl)
              }
            }
            n455 = local read "聚焦值数组"() -> (w917:dbl[])
            n456 = Insert Into Array(array=w917, new element=w916) -> (w918:dbl[])  [unwired: 1 in]
            n457 = local write "聚焦值数组"(w918) -> ()
            n458 = Greater?(x=w919, y=w920) -> (0:w927:bool)
            n459 = Greater?(x=w921, y=w919) -> (0:w924:bool)
            n460 = Boolean To (0,1)(Boolean=w924) -> (0, 1=w923:i16)
            n461 = Boolean To (0,1)(Boolean=w927) -> (0, 1=w922:i16)
            n462 = Multiply(x=i16 10, y=w923) -> (x*y=w925:i16)
            n463 = Add(x=w925, y=w922) -> (x+y=w915:i16)
            "x+y 2" <- w915
            n464 = case shown="11, 默认" w915 {
              tunnel: w914 -> [w929 w938 w953 w957]
              tunnel: [w928 w937 w949 w956] -> w913
              frame 10 {
                # "4继续向上运动"
                n465 = flat-sequence {
                  tunnel: [w935] -> w928
                  tunnel: w929 -> [w934]
                  frame #0 {
                    n466 = local read "变量"() -> (w932:dbl)
                    n467 = Multiply(x=1.0 ("Z 2"), y=w932) -> (x*y=w930:dbl)
                    n468 = call "285A_RelMove.vi"("VISA资源名称"=w934, "Z 2"=w930, "Y 2"=0.0, "X 2"=0.0) -> ("VISA resource name out 2"=w935:refnum<visa-resource-name>)  [unwired: 2 in, 5 out]
                  }
                }
              }
              frame 0 {
                # "2向回运动"
                n469 = flat-sequence {
                  tunnel: w938 -> [w948]
                  tunnel: [w947] -> w937
                  frame #0 {
                    n470 = local read "变量"() -> (w941:dbl)
                    n471 = Multiply(x=-1.0 ("y"), y=w941) -> (x*y=w939:dbl)
                    n472 = local write "变量"(w939) -> ()
                  }
                  frame #1 {
                    n473 = local read "变量"() -> (w944:dbl)
                    n474 = Multiply(x=1.0, y=w944) -> (x*y=w942:dbl)
                    n475 = call "285A_RelMove.vi"("VISA资源名称"=w948, "Z 2"=w942, "Y 2"=0.0, "X 2"=0.0) -> ("VISA resource name out 2"=w947:refnum<visa-resource-name>)  [unwired: 2 in, 5 out]
                  }
                }
              }
              frame 11, Default {
                # "1往上运动"
                n476 = local read "变量"() -> (w951:dbl)
                n477 = Multiply(x=1.0 ("Z 2"), y=w951) -> (x*y=w950:dbl)
                n478 = call "285A_RelMove.vi"("VISA资源名称"=w953, "Z 2"=w950, "Y 2"=0.0, "X 2"=0.0) -> ("VISA resource name out 2"=w949:refnum<visa-resource-name>)  [unwired: 2 in, 5 out]
              }
              frame 1 {
                # "3最大值停止运动"
                n479 = local read "聚焦值数组"() -> (w963:dbl[])
                n480 = Array Max & Min(array=w963) -> (max value=w962:dbl)  [unwired: 3 out]
                n481 = local read "Right"() -> (w959:dbl)
                n482 = Subtract(x=w962, y=6.0) -> (x-y=w960:dbl)
                n483 = Greater?(x=w959, y=w960) -> (0:w958:bool)
                n484 = case shown="假" w958 {
                  tunnel: w957 -> [w968 w971]
                  tunnel: [w964 w971] -> w956
                  frame False {
                    n485 = local read "变量"() -> (w965:dbl)
                    n486 = Multiply(x=3.0 ("Z 2"), y=w965) -> (x*y=w967:dbl)
                    n487 = call "285A_RelMove.vi"("VISA资源名称"=w968, "Z 2"=w967, "Y 2"=0.0, "X 2"=0.0) -> ("VISA resource name out 2"=w964:refnum<visa-resource-name>)  [unwired: 2 in, 5 out]
                  }
                  frame True {
                    n488 = local write "针尖粗对焦"(FALSE ("针尖粗对焦")) -> ()
                  }
                }
              }
            }
          }
        }
      }
      frame #2 {
        n489 = local read "是否匹配到？"() -> (w985:bool)
        n490 = And(x=w985, y="针尖细对焦") -> (x .and. y?=w988:bool)
        n491 = case shown="真" w988 {
          tunnel: w987 -> [w991 w998]
          tunnel: [w991 w997] -> w986
          frame False {
            n492 = local write "针尖细对焦"(FALSE ("针尖细对焦")) -> ()
          }
          frame True {
            n493 = local read "变量"() -> (w994:dbl)
            n494 = Multiply(x=-1.0, y=w994) -> (x*y=w992:dbl)
            n495 = call "285A_RelMove.vi"("VISA资源名称"=w998, "Z 2"=w992, "Y 2"=0.0, "X 2"=0.0) -> ("VISA resource name out 2"=w997:refnum<visa-resource-name>)  [unwired: 2 in, 5 out]
          }
        }
      }
    }
    n496 = local read "针尖坐标"() -> (w806:sgl[])
    n497 = local read "目标坐标"() -> (w807:i32[])
    n498 = case shown="真" "针尖自动移动" {
      tunnel: w808 -> [w855 w878]
      tunnel: [w855 w865] -> w797
      tunnel: w807 -> [_ w867]
      tunnel: w806 -> [_ w860]
      frame False {
      }
      frame True {
        # "模板针尖偏移量"
        # "PID控制针尖移动"
        # "可以直接用pid模块"
        n499 = Index Array(array=w860, index=1 ("索引")) -> (element=w857:sgl)
        n500 = Index Array(array=w860, index=0 ("索引")) -> (element=w856:sgl)
        n501 = Index Array(array=w867, index=1 ("索引")) -> (element=w876:i32)
        n502 = Index Array(array=w867, index=0 ("索引")) -> (element=w877:i32)
        n503 = Subtract(x=w876, y=w857) -> (x-y=w872:sgl)
        n504 = Bundle("x"=w857, w876) -> ()  [unwired: 1 in, 1 out]
        n505 = Add(x=sgl 0.0 ("y"), y=w856) -> (x+y=w861:sgl)
        n506 = Subtract(x=w877, y=w861) -> (x-y=w873:sgl)
        n507 = call-poly <vilib>:"PID.vi"("PID gains"="PID gains", "process variable"=w861, "setpoint"=w877) -> ("output"=w863:dbl)  [unwired: 7 in, 1 out]
        n508 = call-poly <vilib>:"PID.vi"("PID gains"="PID gains 2", "process variable"=w857, "setpoint"=w876) -> ("output"=w864:dbl)  [unwired: 7 in, 1 out]
        n509 = Bundle("x"=w856, w877) -> ()  [unwired: 1 in, 1 out]
        n510 = Square(x=w873) -> (x^2=w871:sgl)
        n511 = Square(x=w872) -> (x^2=w870:sgl)
        n512 = Add(x=w871, y=w870) -> (x+y=w866:sgl)
        n513 = Greater?(x=w866, y=15.0) -> (0:w879:bool)
        n514 = case shown="真" w879 {
          tunnel: w878 -> [w883 w887]
          tunnel: [w883 w886] -> w865
          tunnel: w863 -> [_ w885]
          tunnel: w864 -> [_ w884]
          frame False {
            n515 = local write "针尖自动移动"(FALSE) -> ()
            n516 = One Button Dialog(message="针尖已移动到目标位置" ("消息")) -> ()  [unwired: 1 in, 1 out]
          }
          frame True {
            # "阈值范围需要调整，太大针尖检测不出来，太小程序会出现bug'"
            n517 = flat-sequence {
              tunnel: w887 -> [w894]
              tunnel: [w893] -> w886
              tunnel: w885 -> [w889]
              tunnel: w884 -> [w888]
              frame #0 {
                # "x位置p负号原因是设备转换后的"
                n518 = To Byte Integer(number=w888) -> (8bit integer=w892:i8)
                n519 = To Byte Integer(number=w889) -> (8bit integer=w891:i8)
                n520 = In Range and Coerce(upper limit=2.0 ("上限"), x=w892, lower limit=-2.0 ("上限")) -> (coerced(x)=w897:dbl)  [unwired: 1 out]
                n521 = In Range and Coerce(upper limit=2.0 ("上限"), x=w891, lower limit=-2.0 ("上限")) -> (coerced(x)=w890:dbl)  [unwired: 1 out]
                n522 = call "285A_RelMove.vi"("VISA资源名称"=w894, "Z 2"=0.0 ("Z"), "Y 2"=w897, "X 2"=w890) -> ("VISA resource name out 2"=w893:refnum<visa-resource-name>)  [unwired: 2 in, 5 out]
              }
            }
          }
        }
      }
    }
    n523 = case shown="真" "自动接触" {
      tunnel: w797 -> [w999 w1008]
      tunnel: [w999 w1003] -> w804
      frame False {
      }
      frame True {
        # "阈值"
        n524 = local read "校准的入液阻值"() -> (w1002:dbl)
        n525 = local read "阻值数组"() -> (w1014:dbl[])
        n526 = Index Array(array=w1014, index=0 ("索引")) -> (element=w1007:dbl)
        n527 = Index Array(array=w1014, index=1 ("索引")) -> (element=w1012:dbl)
        n528 = Index Array(array=w1014, index=2 ("索引")) -> (element=w1011:dbl)
        n529 = Multiply(x=1.01, y=w1002) -> (x*y=w1000:dbl)
        n530 = Greater Or Equal?(x=w1007, y=w1012) -> (x >= y?=w1010:bool)
        n531 = Greater Or Equal?(x=w1012, y=w1011) -> (x >= y?=w1009:bool)
        n532 = Greater?(x=w1007, y=w1000) -> (0:w1006:bool)
        n533 = And(x=w1010, y=w1009) -> (x .and. y?=w1005:bool)
        n534 = And(x=w1006, y=w1005) -> (x .and. y?=w1004:bool)
        n535 = case shown="假" w1004 {
          tunnel: w1008 -> [w1021 w1030]
          tunnel: [w1022 w1030] -> w1003
          frame False {
            # "向下运动"
            n536 = case shown="真" "下降/向右" {
              tunnel: [0.0 ("X 2") "下降步伐/um"] -> w1019
              tunnel: [w1025 0.0 ("X 2")] -> w1018
              tunnel: [0.0 ("Y 2") 0.0 ("Y 2")] -> w1017
              frame False {
                n537 = local read "下降步伐/um"() -> (w1025:dbl)
              }
              frame True {
              }
            }
            n538 = call "285A_RelMove.vi"("VISA资源名称"=w1021, "Z 2"=w1019, "Y 2"=w1017, "X 2"=w1018) -> ("VISA resource name out 2"=w1022:refnum<visa-resource-name>)  [unwired: 2 in, 5 out]
          }
          frame True {
            n539 = local write "自动接触"(FALSE) -> ()
            n540 = One Button Dialog(message="电极已接触细胞" ("消息")) -> ()  [unwired: 1 in, 1 out]
          }
        }
      }
    }
    n541 = case shown="真" "保存数据" {
      tunnel: w804 -> [w838 w854]
      tunnel: [w829 w854] -> w803
      tunnel: w801 -> [w831 w853]
      tunnel: w800 -> [w827 _]
      tunnel: [w830 w853] -> w798
      tunnel: w799 -> [w825 _]
      frame True {
        w821 = "\t"
        n542 = local read "Resistance(MΩ)"() -> (w828:dbl)
        n543 = call "285A_GetPos.vi"("VISA资源名称"=w838) -> ("Z"=w833:dbl, "Y"=w835:dbl, "X"=w837:dbl, "VISA资源名称输出"=w829:refnum<visa-resource-name>)  [unwired: 5 in, 2 out]
        n544 = Quotient & Remainder(x=w825, y=100) -> (x-y*floor(x/y)=w823:i32)  [unwired: 1 out]
        n545 = Get Date/Time String(want seconds? (F)=TRUE ("需要秒？(F)")) -> (time string=w819:string)  [unwired: 2 in, 1 out]
        n546 = Number To Fractional String(number=w835) -> (F-format string=w834:string)  [unwired: 3 in]
        n547 = Number To Decimal String(number=w825) -> (decimal integer string=w826:string)  [unwired: 1 in]
        n548 = Number To Fractional String(number=w837) -> (F-format string=w836:string)  [unwired: 3 in]
        n549 = Number To Fractional String(number=w833) -> (F-format string=w832:string)  [unwired: 3 in]
        n550 = Number To Fractional String(number=w828) -> (F-format string=w844:string)  [unwired: 3 in]
        n551 = Equal?(x=w823, y=0) -> (x = y?=w818:bool)
        n552 = case shown="真" w818 {
          tunnel: w827 -> [_ w848]
          tunnel: w826 -> [_ w846]
          frame False {
          }
          frame True {
            n553 = Concatenate Strings("图像" ("字符串"), w846, ".bmp" ("字符串")) -> (w850:string)
            n554 = local read "Image"() -> (w847:T1)
            n555 = Build Path(base path=w848, name or relative path=w850) -> (appended path=w852:path)
            n556 = call-poly "IMAQ Write File 2"("File Path"=w852, "Image"=w847) -> ()  [unwired: 8 in, 2 out]
          }
        }
        n557 = Concatenate Strings(w819, w821, w826, w821, w821, "X轴：" ("字符串"), w836, w821, "Y轴：" ("字符串"), w834, w821, "Z轴：" ("字符串"), w832, w821, "阻值：" ("字符串"), w844, "\n") -> (w839:string)
        n558 = Write to Text File(file (use dialog)=w831, text=w839) -> (refnum out=w830:refnum<file>)  [unwired: 2 in, 2 out]
      }
      frame False {
      }
    }
  }
  n559 = Boolean Array To Number(Boolean array=w59) -> (number=w60:u32)
  n560 = call "SetDA.vi"("错误输入（无错误）"=w68, "DAVolt"=0.0, "DANum"=u8 3, "DevIndex"=w69) -> ("错误输出"=w55:errorcluster, "DevIndex Output"=w56:i32)  [unwired: 6 in]
  n561 = To Unsigned Byte Integer(number=w60) -> (unsigned 8bit integer=w58:u8)
  n562 = call "SetDioOut.vi"("错误输入（无错误）"=w55, "DioOut"=w58, "DioChanSel"=u8 255, "DevIndex"=w56) -> ("错误输出"=w54:errorcluster, "DevIndex Output"=w53:i32)  [unwired: 6 in]
  n563 = call "StopRead.vi"("错误输入（无错误）"=w54, "DevIndex"=w53) -> ("错误输出"=w79:errorcluster, "DevIndex Output"=w80:i32)  [unwired: 8 in]
  n564 = call "Imaq Dispose"("Image"=w107, "error in (no error)"=w106) -> ("error out"=w112:errorcluster)  [unwired: 4 in]
  n565 = call <vilib>:"IMAQdx Close Camera.vi"("error in"=w104, "Session In"=w111) -> ("error out"=w113:errorcluster)  [unwired: 9 in]
  n566 = call "SetSoftTrig.vi"("错误输入（无错误）"=w79, "Trig"=u8 0, "DevIndex"=w80) -> ("错误输出"=w78:errorcluster, "DevIndex Output"=w76:i32)  [unwired: 7 in]
  n567 = Release Queue(queue=w101, error in (no error)=w100) -> (error out=w51:errorcluster)  [unwired: 1 in, 2 out]
  n568 = call "ClearTrigger.vi"("错误输入（无错误）"=w78, "DevIndex"=w76) -> ("错误输出"=w77:errorcluster, "DevIndex Output"=w75:i32)  [unwired: 8 in]
  n569 = Merge Errors(w112, w113, w51) -> (→"错误输出":errorcluster)
  n570 = call "ClearBufs.vi"("错误输入（无错误）"=w77, "DevIndex"=w75) -> ("错误输出"=w81:errorcluster, "DevIndex Output"=w82:i32)  [unwired: 8 in]
  n571 = call "CloseDevice.vi"("错误输入（无错误）"=w81, "DevIndex"=w82) -> ("错误输出"=w38:errorcluster)  [unwired: 8 in, 1 out]
  n572 = Merge Errors(w39, w38) -> (→"错误输出 3":errorcluster)
  n573 = Close File(refnum=w22) -> ()  [unwired: 1 in, 2 out]
  n574 = call "285A_Update.vi"("VISA资源名称"=w37) -> ("VISA资源名称 2"=w40:refnum<visa-resource-name>)  [unwired: 9 in, 1 out]
  n575 = VISA Close(VISA resource name=w40) -> ()  [unwired: 1 in, 1 out]
